vi "北控main.vi"() -> ()   [LabVIEW 2015]
uses:
  <vilib>/addons/database/Connection.llb/Conn ObjectReference.ctl
  <vilib>/addons/database/Auxilliary.llb/DB Tools Column Info.ctl
  <vilib>/addons/database/Auxilliary.llb/DB Tools DataTypes.ctl
  ModbusRTU/bin/Debug/Advantech.Adam.dll
  <vilib>/Instr/_visa.llb/VISA Flush IO Buffer Mask.ctl
  <vilib>/Utility/config.llb/Read Key (String).vi
  <vilib>/Utility/config.llb/Read Key (I32).vi
  <vilib>/Utility/config.llb/Read Key (Double).vi
  <vilib>/Instr/_visa.llb/VISA Configure Serial Port (Instr).vi
  <vilib>/Utility/config.llb/Write Key (String).vi
  <vilib>/Utility/config.llb/Write Key (I32).vi
  <vilib>/Utility/config.llb/Write Key (Double).vi
  <vilib>/regexp/Match Regular Expression.xnode
  <vilib>/addons/database/NI_Database_API.lvlib
  <vilib>/Utility/config.llb/NI_LVConfig.lvlib
panel:
  out "P1.0":dbl format="%#.3f"
  out "P2.0":dbl format="%#.3f"
  out "ISCOTCP":refnum<k5>
  in  "PressureCardID":i32=3
  out "adam串口正常":bool
  out "adamcom":refnum<k24>
  out "adammodbus":refnum<k24>
  out "TCPSuspend":bool
  in  "Adjust":dbl
  in  "WaterSeperation1.0":dbl
  in  "OilSeperation1.0":dbl
  out "OilValueCal":bool
  out "WaterValueCal":bool
  in  "PreOilValue":dbl
  in  "PreWaterValue":dbl
  out "ICControl":refnum<k7>
  out "YRDTCP":refnum<k5>
  out "Mettler VISA":refnum<visa-resource-name> caption="VISA资源名称输出"
  out "Mettler串口正常":bool
  in  "column information":T1=[{"column name"="RecordingTime", "data type"=enum."String", "size"=50, "allow null?"=TRUE}, {"column name"="CumulativeOilProduction", "data type"=enum."Double (DBL)", "size"=0, "allow null?"=TRUE}, {"column name"="CumulativeWaterProduction", "data type"=enum."Double (DBL)", "size"=0, "allow null?"=TRUE}, {"column name"="BalanceValue", "data type"=enum."Double (DBL)", "size"=0, "allow null?"=TRUE}, {"column name"="DifferencialPressure", "data type"=enum."Double (DBL)", "size"=0, "allow null?"=TRUE}, {"column name"="Pressure1", "data type"=enum."Double (DBL)", "size"=0, "allow null?"=TRUE}, {"column name"="Pressure2", "data type"=enum."Double (DBL)", "size"=0, "allow null?"=TRUE}, {"column name"="CPPOuterPre", "data type"=enum."Double (DBL)", "size"=0, "allow null?"=TRUE}, {"column name"="CPPTracePre", "data type"=enum."Double (DBL)", "size"=0, "allow null?"=TRUE}, {"column name"="CPPCurrentVol", "data type"=enum."Double (DBL)", "size"=0, "allow null?"=TRUE}, {"column name"="CPPInnerPre", "data type"=enum."Double (DBL)", "size"=0, "allow null?"=TRUE}, {"column name"="FlowSetpointA", "data type"=enum."Double (DBL)", "size"=0, "allow null?"=TRUE}, {"column name"="PressureSetpointA", "data type"=enum."Double (DBL)", "size"=0, "allow null?"=TRUE}, {"column name"="FlowRateA", "data type"=enum."Double (DBL)", "size"=0, "allow null?"=TRUE}, {"column name"="PressuerA", "data type"=enum."Double (DBL)", "size"=0, "allow null?"=TRUE}, {"column name"="FlowSetpointB", "data type"=enum."Double (DBL)", "size"=0, "allow null?"=TRUE}, {"column name"="PressureSetpointB", "data type"=enum."Double (DBL)", "size"=0, "allow null?"=TRUE}, {"column name"="FlowRateB", "data type"=enum."Double (DBL)", "size"=0, "allow null?"=TRUE}, {"column name"="PressuerB", "data type"=enum."Double (DBL)", "size"=0, "allow null?"=TRUE}, {"column name"="InspectionItem", "data type"=enum."String", "size"=0, "allow null?"=TRUE}, {"column name"="WellNumber", "data type"=enum."String", "size"=0, "allow null?"=TRUE}, {"column name"="DateofExperiment", "data type"=enum."String", "size"=0, "allow null?"=TRUE}, {"column name"="NumberofSample", "data type"=enum."String", "size"=0, "allow null?"=TRUE}, {"column name"="LithologicalCharacter ", "data type"=enum."String", "size"=0, "allow null?"=TRUE}, {"column name"="ExperimentalTemperature ", "data type"=enum."String", "size"=0, "allow null?"=TRUE}, {"column name"="SimulatedOilViscosity ", "data type"=enum."String", "size"=0, "allow null?"=TRUE}, {"column name"="InjectionWaterViscosity", "data type"=enum."String", "size"=0, "allow null?"=TRUE}, {"column name"="LengthofRockSample", "data type"=enum."String", "size"=0, "allow null?"=TRUE}, {"column name"="PoreVolume ", "data type"=enum."String", "size"=0, "allow null?"=TRUE}, {"column name"="CoreDepth ", "data type"=enum."String", "size"=0, "allow null?"=TRUE}, {"column name"="AirPermeability ", "data type"=enum."String", "size"=0, "allow null?"=TRUE}, {"column name"="SimulatedOilDensity", "data type"=enum."String", "size"=0, "allow null?"=TRUE}, {"column name"="InjectionWaterDensity", "data type"=enum."String", "size"=0, "allow null?"=TRUE}, {"column name"="RockSampleDiameter ", "data type"=enum."String", "size"=0, "allow null?"=TRUE}, {"column name"="Porosity", "data type"=enum."String", "size"=0, "allow null?"=TRUE}, {"column name"="InletPressure", "data type"=enum."String", "size"=0, "allow null?"=TRUE}, {"column name"="OutletPressure", "data type"=enum."String", "size"=0, "allow null?"=TRUE}, {"column name"="IrreducibleWaterSaturation", "data type"=enum."String", "size"=0, "allow null?"=TRUE}, {"column name"="SectionalArea", "data type"=enum."String", "size"=0, "allow null?"=TRUE}, {"column name"="VolumeOfRockSample", "data type"=enum."String", "size"=0, "allow null?"=TRUE}]
  out "Suspend":dbl
  out "Stop":dbl
  in  "选项卡控件":T4(tab)
  in  "压力校零":bool
  out "Pressure Setpoint B":dbl
  out "Flow Setpoint B":dbl
  out "Pressure Setpoint A":dbl
  out "Flow Setpoint A":dbl
  out "Pressure B":dbl
  out "Pressure A":dbl
  out "Flow Rate B":dbl
  out "Flow Rate A":dbl
  out "液罐 18":dbl(slide) scale=0.0..10.0
  out "液罐 26":dbl(slide) scale=0.0..10.0
  out "压差曲线":dbl(graph)
  out "压力曲线":cluster{"P1":dbl, "P2":dbl}(graph)
  out "布尔 157":bool
  in  "Mode Selection":u16(ring) items=["Oil-Water", "Oil-Gas"]
  out "液罐 9":dbl(slide) scale=0.0..10.0
  out "液罐 20":dbl(slide)=9.23076923076923 scale=0.0..10.0
  out "布尔 243":bool
  out "布尔 242":bool=TRUE
  in  "WaterValueCanlibration":bool
  out "WaterValue":dbl format="%#.3f"
  out "OilValue":dbl format="%#.3f"
  in  "OilValueCanlibration":bool
  out "DIF1":dbl format="%#.3g"
  out "P2(夹持器后端)":dbl format="%#.3f"
  out "液罐 17":dbl(slide) scale=0.0..10.0
  in  "DifPressure Canlibration":bool
  out "布尔 240":bool
  out "布尔 24":bool
  out "液罐 7":dbl(slide) scale=0.0..10.0
  out "布尔 6":bool
  out "液罐 6":dbl(slide) scale=0.0..10.0
  out "布尔 5":bool
  out "布尔 4":bool
  in  "btnExit":bool
  out "Weight":dbl format="%#.3f"
  out "布尔 8":bool
  out "布尔 25":bool
  out "液罐 10":dbl(slide) scale=0.0..10.0
  out "液罐 12":dbl(slide) scale=0.0..10.0
  out "液罐 13":dbl(slide) scale=0.0..10.0
  out "液罐 15":dbl(slide) scale=0.0..10.0
  out "液罐 16":dbl(slide) scale=0.0..10.0
  out "布尔 156":bool
  out "布尔 226":bool
  in  "灌泵":bool
  in  "打开跟踪泵":bool
  in  "SetDif(MPa)":dbl
  in  "SetPressure(MPa)":dbl
  in  "TraceMode":enum16{"TraceOuterPre", "TraceSetPre"}(ring)
  out "Suction":bool
  out "Drainage":bool
  in  "清泵":bool
  in  "关闭跟踪泵":bool
  out "CurrentVol(ml)":dbl format="%#.3g"
  out "InnerPre(MPa)":dbl format="%#.3g"
  out "TracePre(MPa)":dbl format="%#.3g"
  out "OuterPre(MPa)":dbl format="%#.3g"
  in  "SetVol(ml)":dbl
  in  "SafePre(MPa)":dbl
  out "P1(夹持器前端)":dbl format="%#.3f"
  in  "DocumentName":string
  in  "开始记录":bool
  in  "数值输入控件":dbl=2.0
  in  "文本下拉列表":u16(ring) items=["second", "minute"]
  out "Number":i32
  out "h":i64
  out "m":i32
  out "s":i32
  in  "停止记录":bool
  in  "暂停记录":bool
  in  "Change Document Name":bool
  in  "MettlerID":refnum<visa-resource-name>="COM11" caption="Mettler串口号"
  out "?":picture
  out "StartSaving":bool
  in  "ICImagingControl":refnum<k7>(container)
  out "数据库文件名":string
  out "DataBase":T5
  # "DataSaveConfiguration"
  # "DataSaveTimeInterval"
  # "psi"
  # "psi"
  # "psi"
  # "g"
  # "oil"
  # "oil"
  # "PMHP01"
  # "water"
  # "water"
  # "ml"
  # "Manual\n Pump"
  # "ml"
  # "BPV"
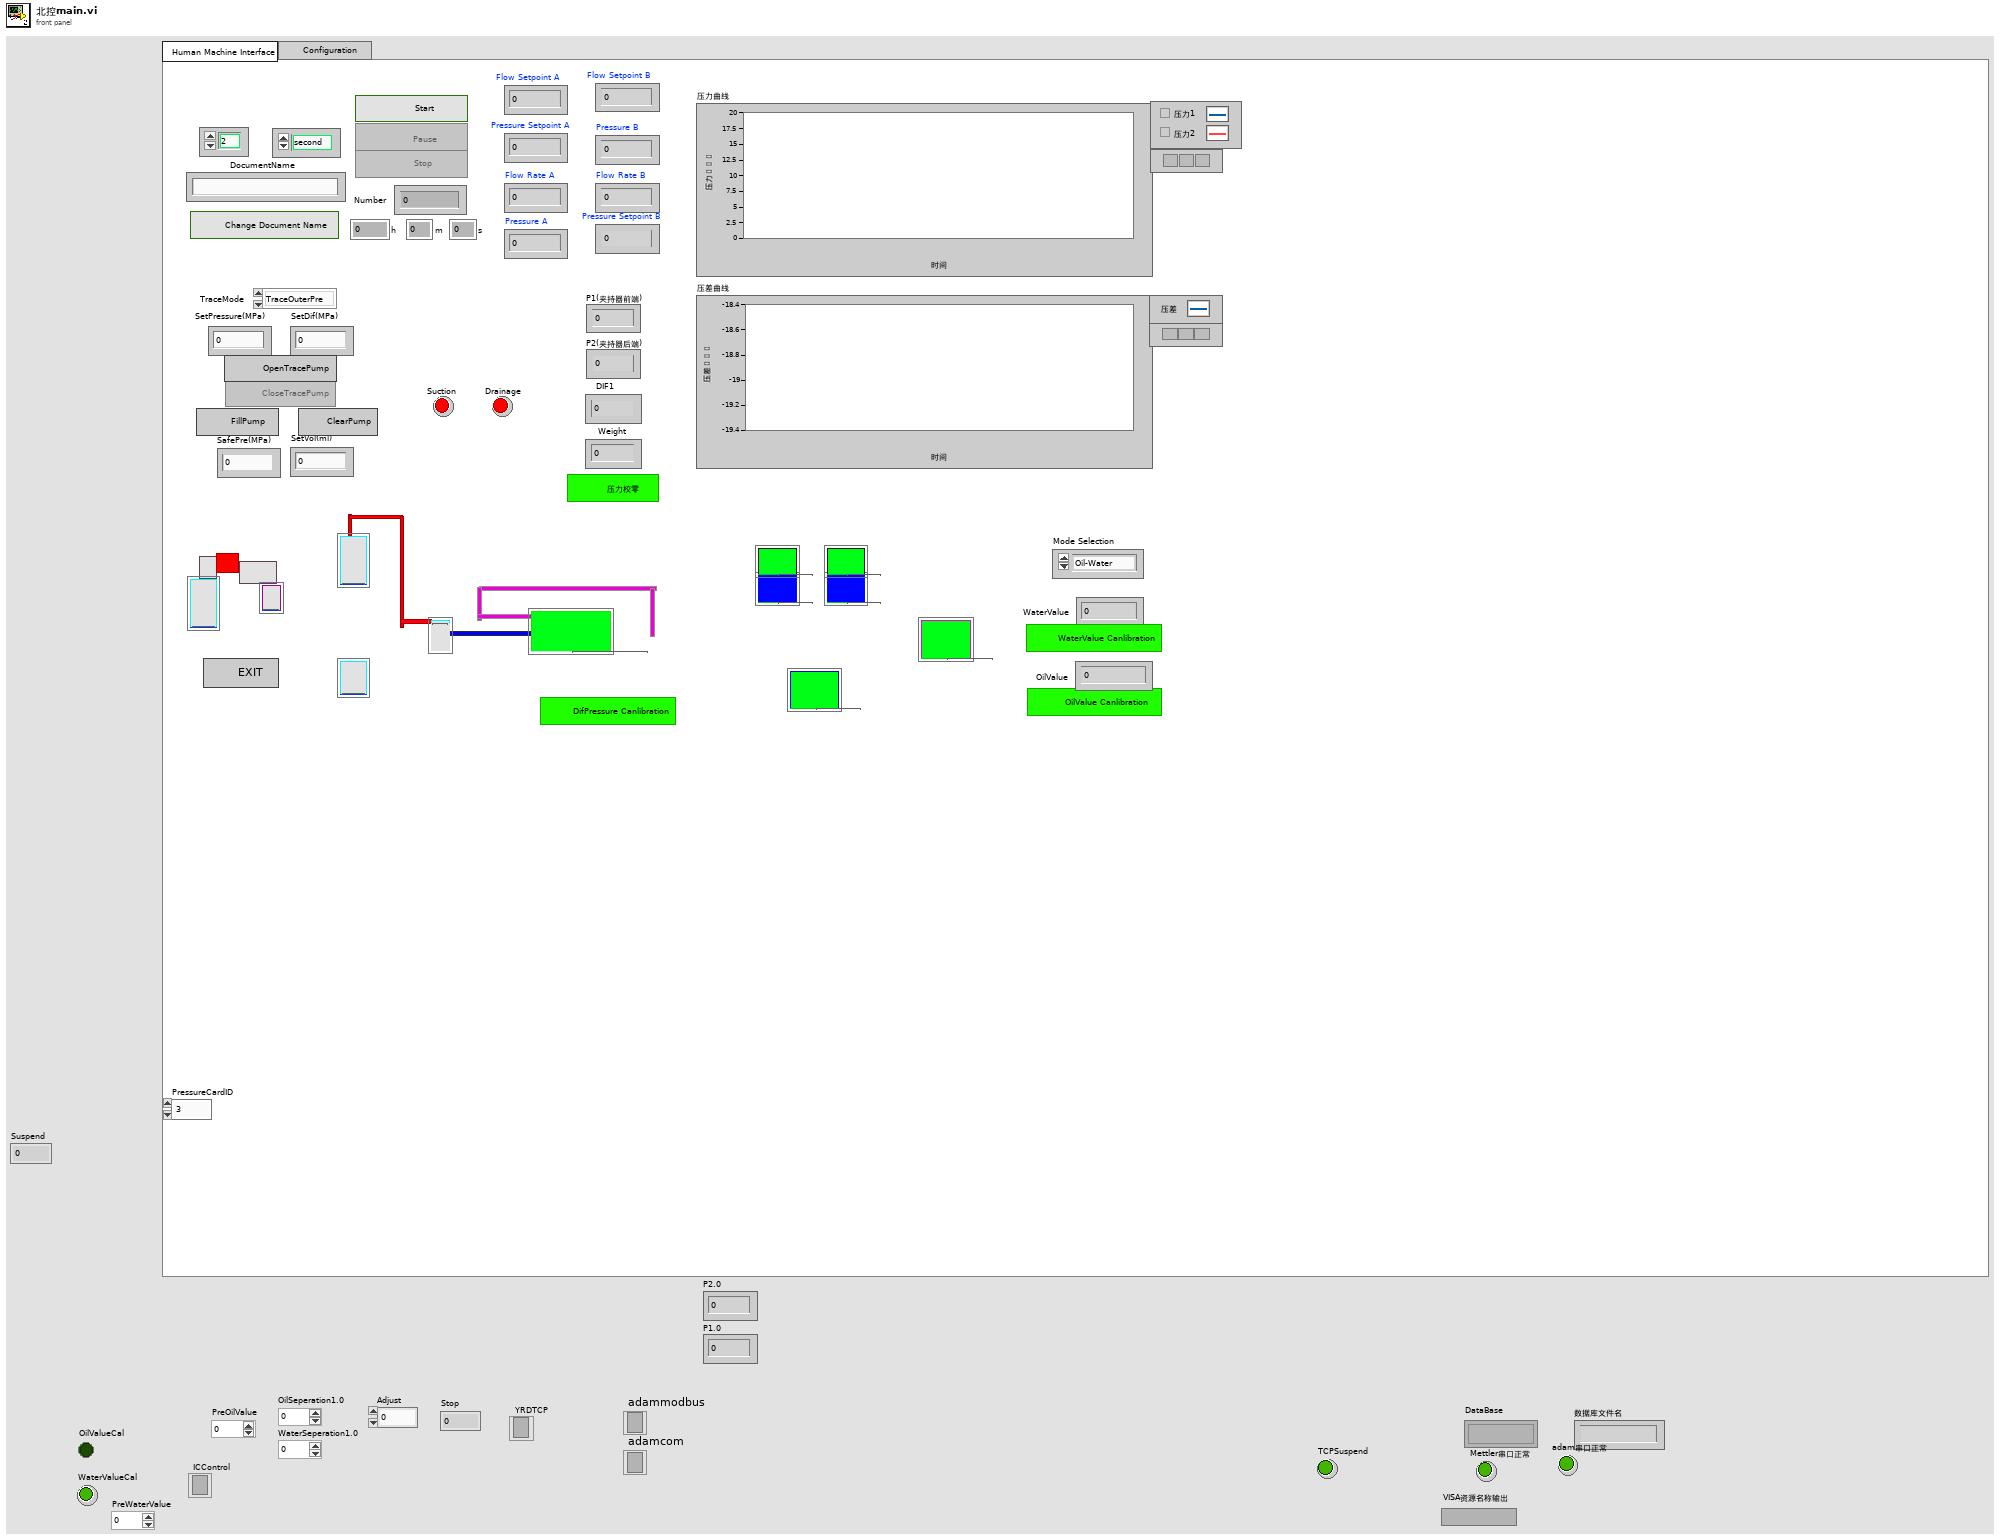
[diagram p1: front panel]
types:
  T1 = typedef "控件 1.ctl" = T2[]
  T2 = typedef "NI_Database_API.lvlib/DB Tools Column Info.ctl" = cluster{"column name":string, "data type":T3, "size":i32, "allow null?":bool}
  T3 = typedef "NI_Database_API.lvlib/DB Tools DataTypes.ctl" = enum16{"String", "Long (I32)", "Single (SGL)", "Double (DBL)", "Date/Time", "Binary"}
  T4 = enum32{" Human Machine Interface  ", "  Configuration            "}
  T5 = typedef "NI_Database_API.lvlib/Conn ObjectReference.ctl" = refnum<k1>
  T6 = enum8{"Enabled", "Disabled", "Disabled and Grayed Out"}
  T7 = typedef "NI_LVConfig.lvlib/Config Data RefNum.ctl" = refnum<k1>
  T8 = typedef "VISA Flush IO Buffer Mask.ctl" = u16
  T9 = cluster{string, "OilValue":dbl, "WaterValue":dbl, "Weight":dbl, "DIF1":dbl, "P1(夹持器前端)":dbl, "P2(夹持器后端)":dbl, "OuterPre(MPa)":dbl, "TracePre(MPa)":dbl, "CurrentVol(ml)":dbl, "InnerPre(MPa)":dbl, "Flow Setpoint A":dbl, "Pressure Setpoint A":dbl, "Flow Rate A":dbl, "Pressure A":dbl, "Flow Setpoint B":dbl, "Pressure Setpoint B":dbl, "Flow Rate B":dbl, "Pressure B":dbl}
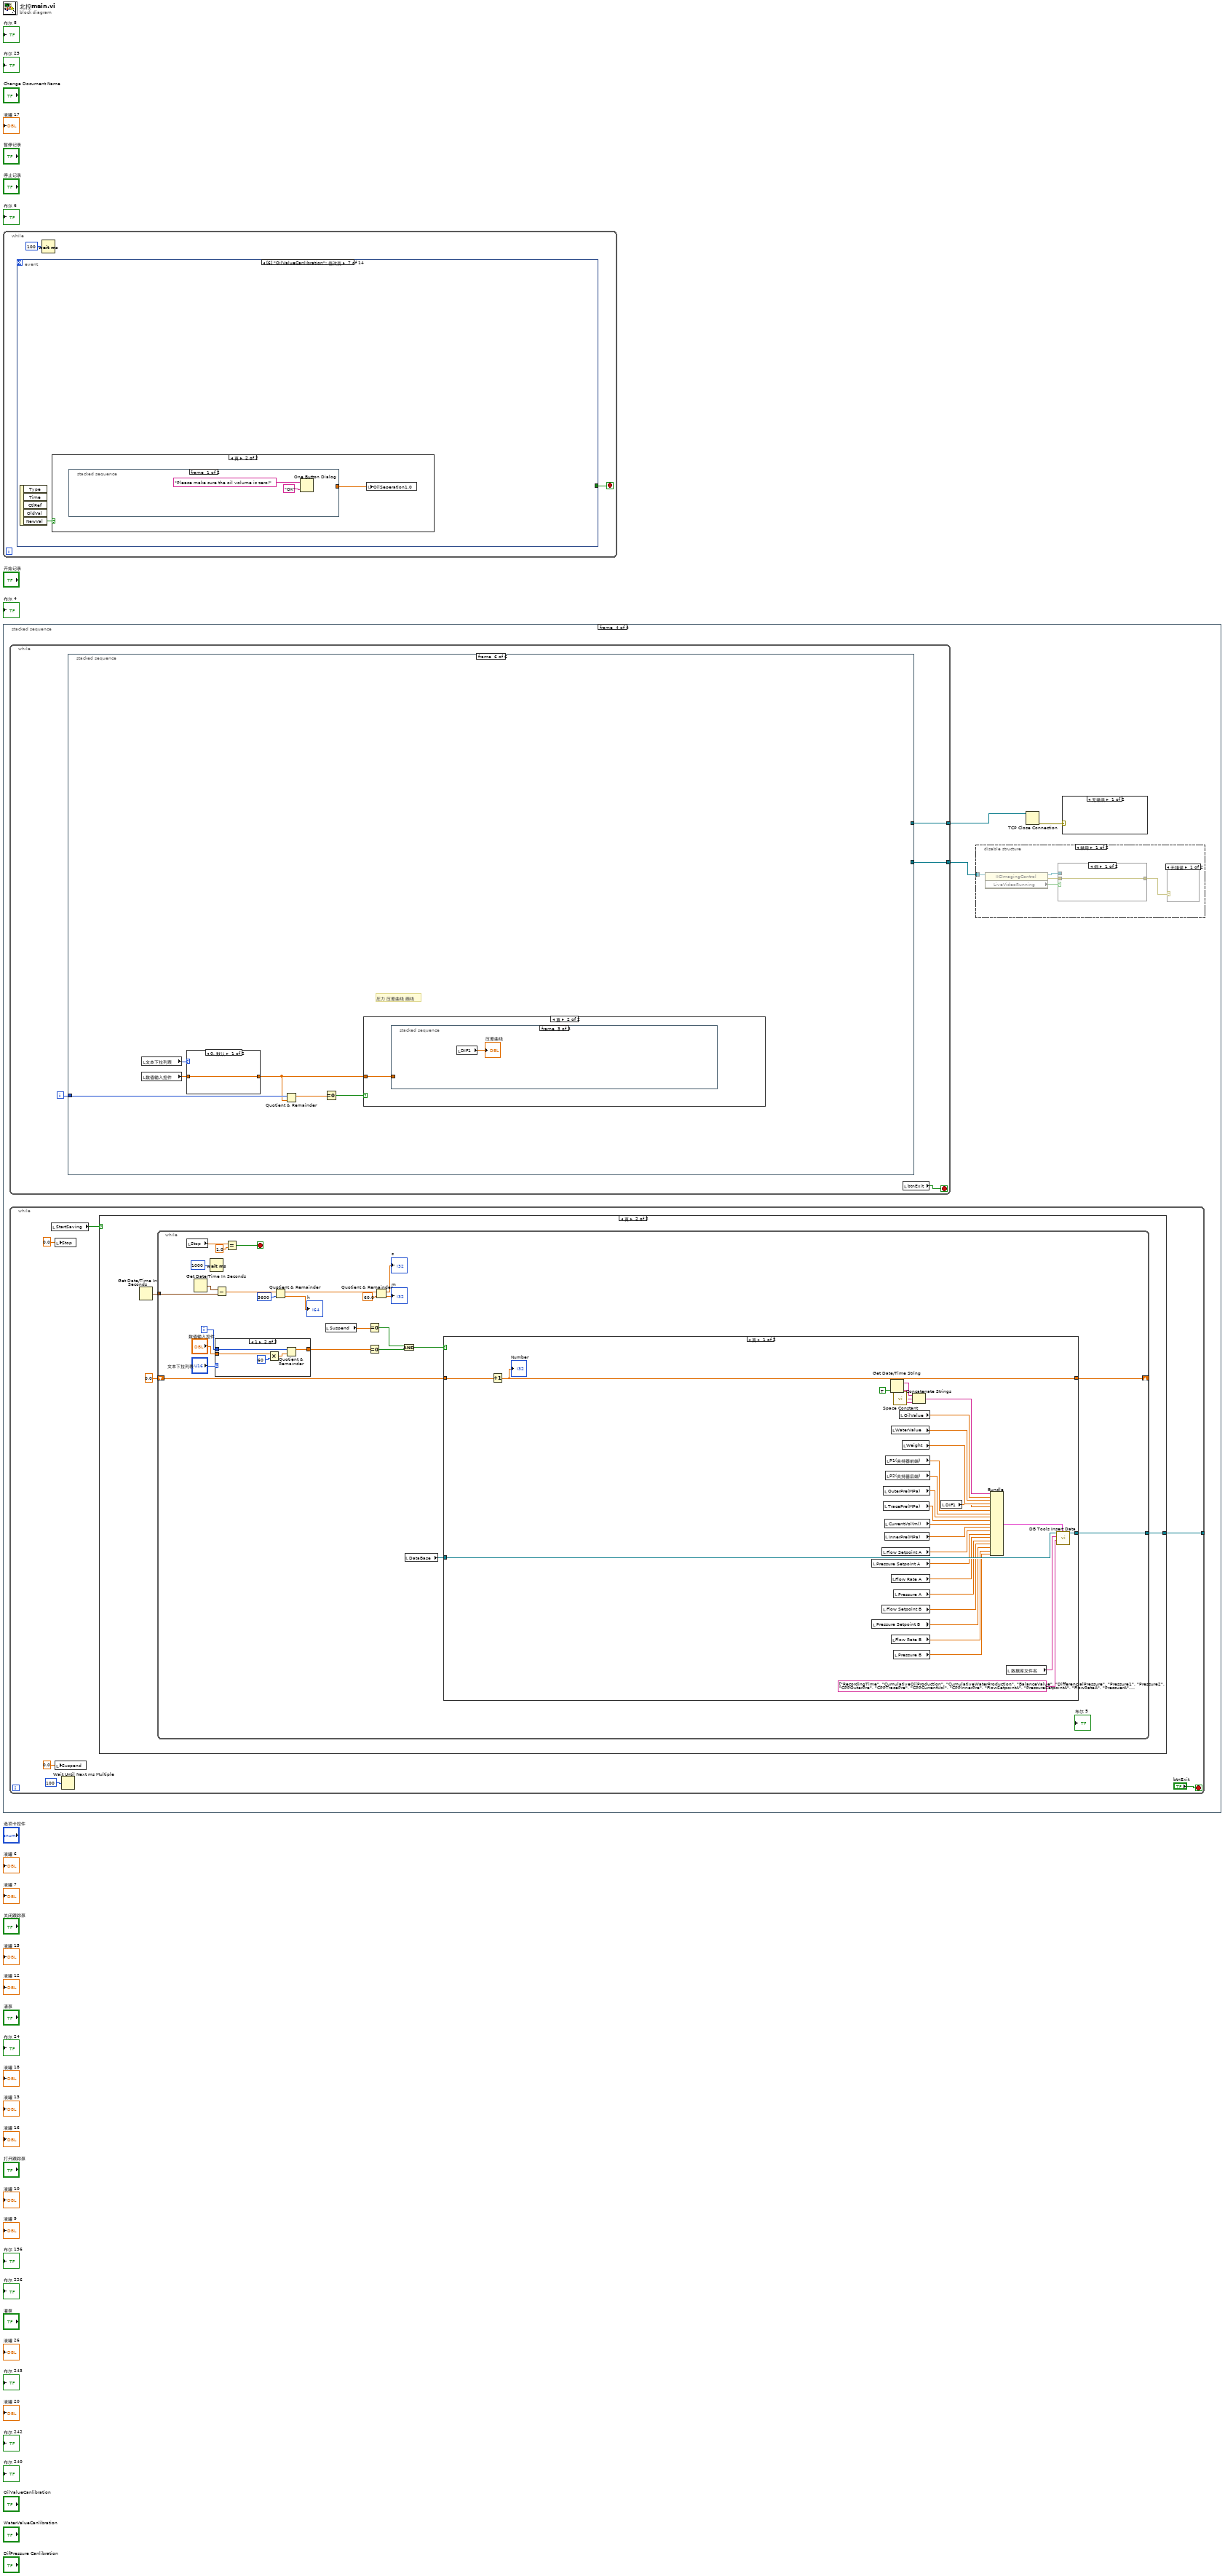
[diagram p0: block diagram]
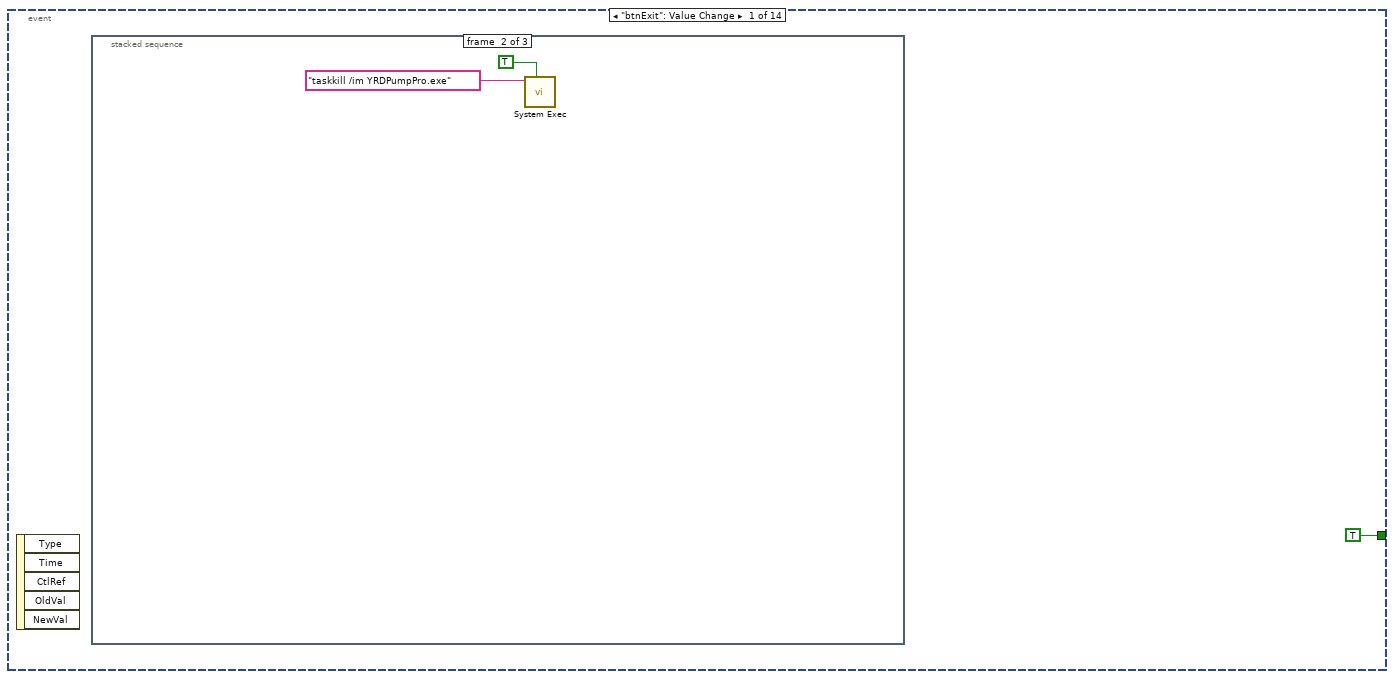
[diagram p2: hidden frame]
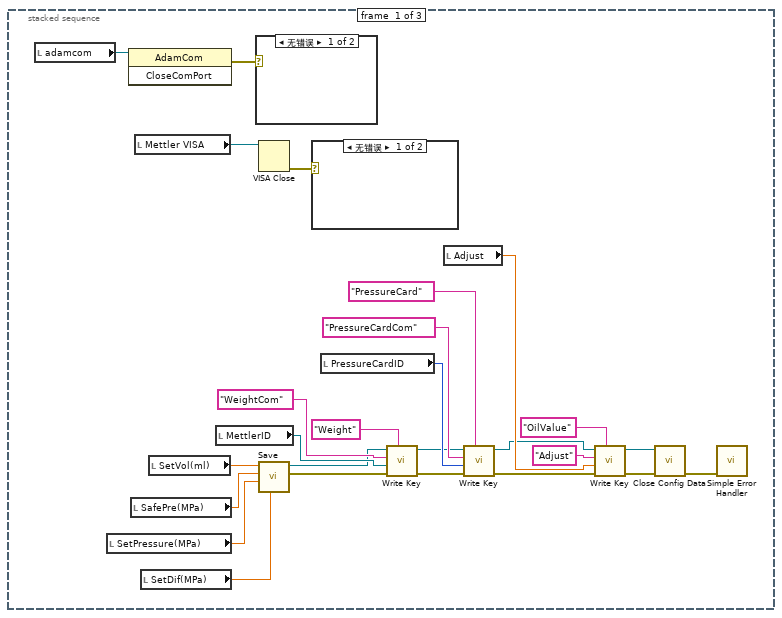
[diagram p3: hidden frame]
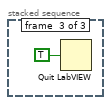
[diagram p6: hidden frame]
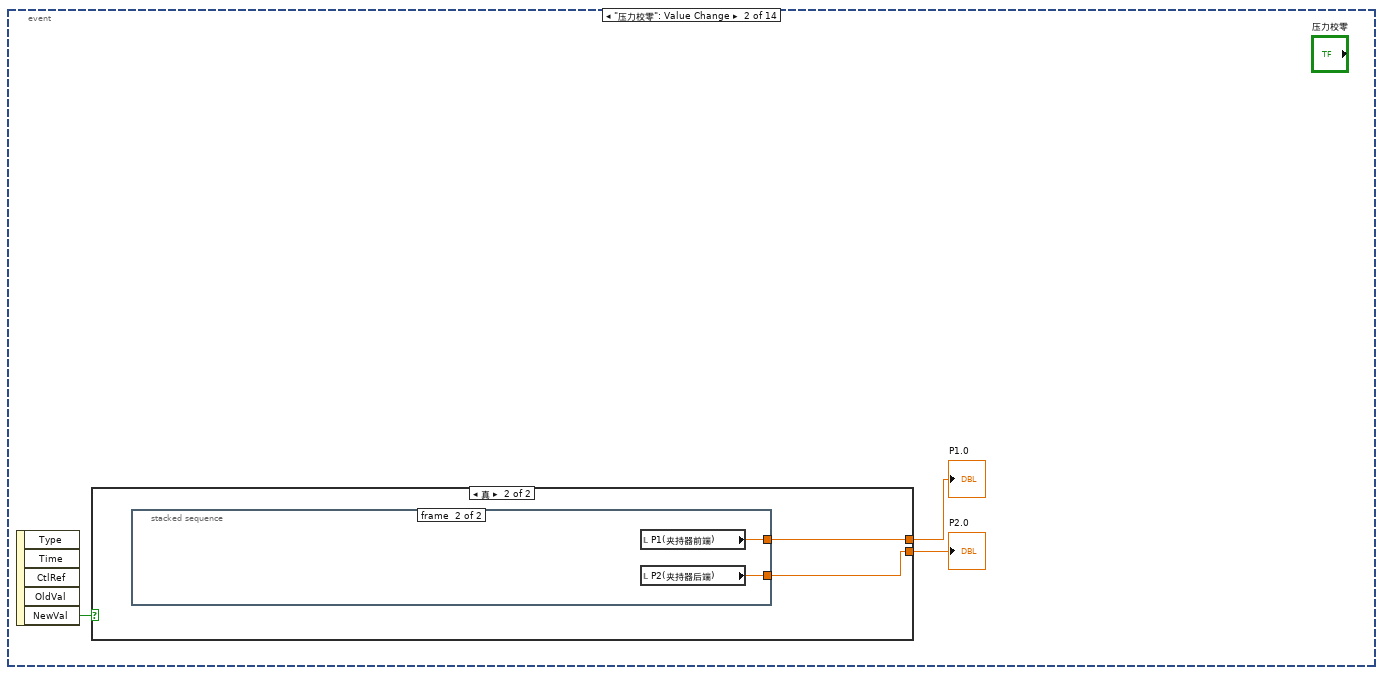
[diagram p7: hidden frame]
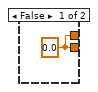
[diagram p8: hidden frame]
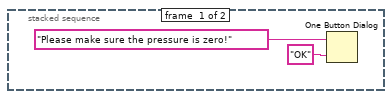
[diagram p9: hidden frame]
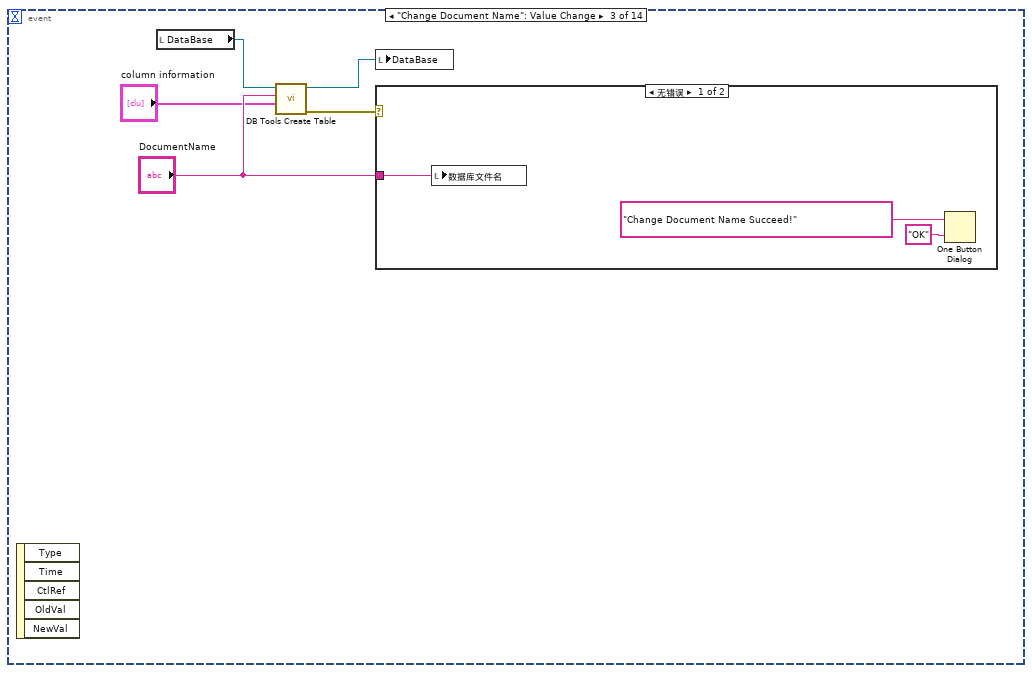
[diagram p10: hidden frame]
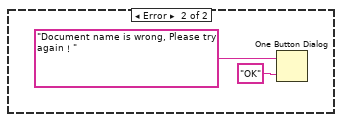
[diagram p11: hidden frame]
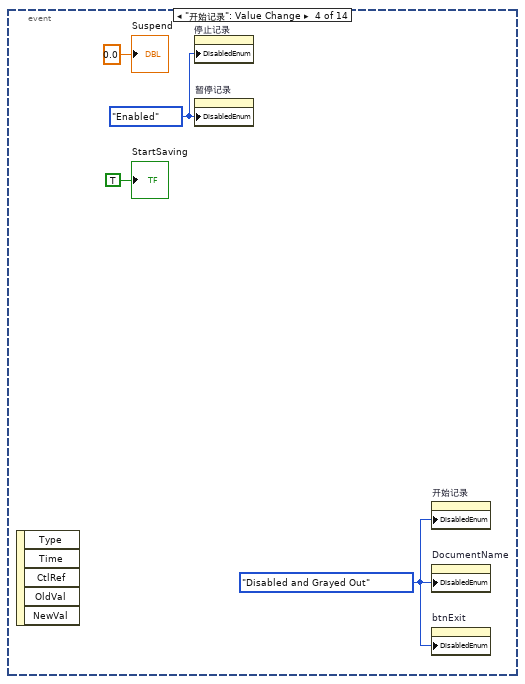
[diagram p12: hidden frame]
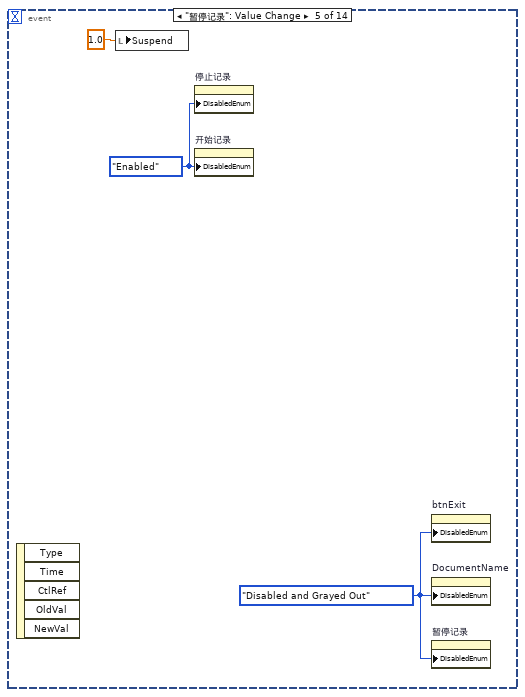
[diagram p13: hidden frame]
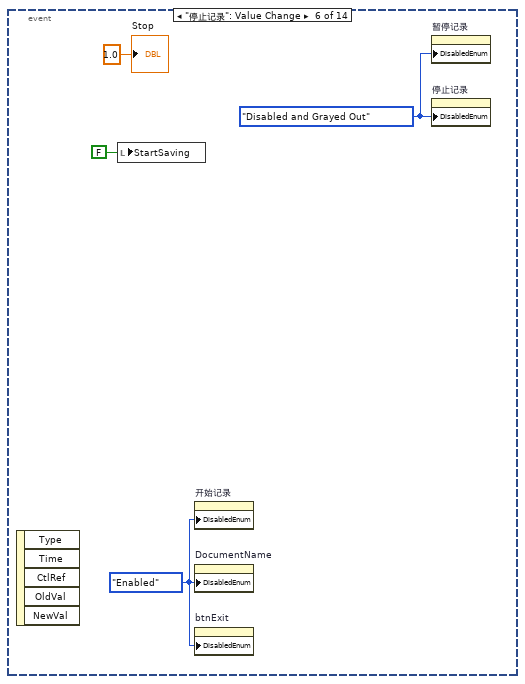
[diagram p14: hidden frame]
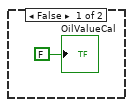
[diagram p15: hidden frame]
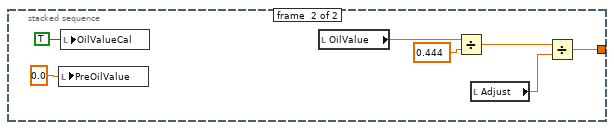
[diagram p16: hidden frame]
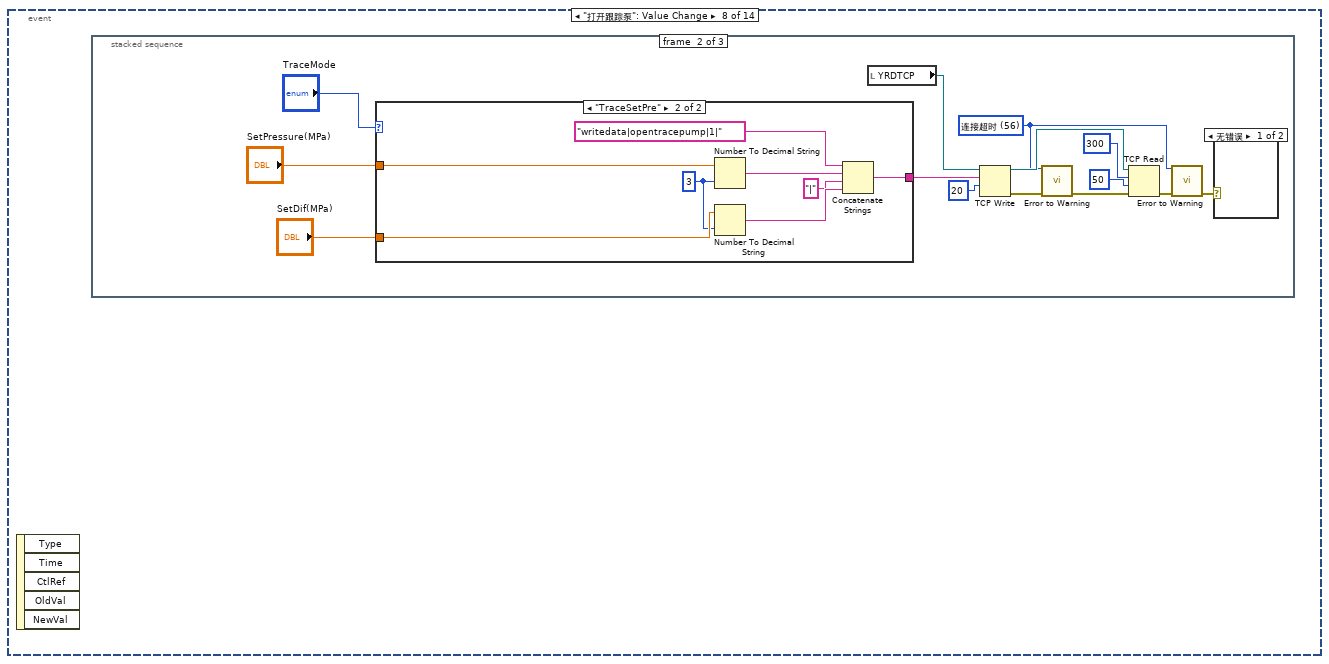
[diagram p17: hidden frame]
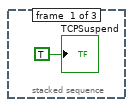
[diagram p18: hidden frame]
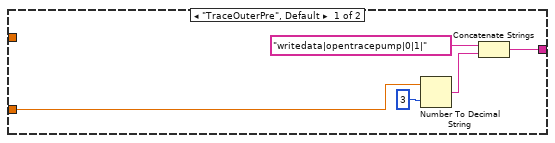
[diagram p20: hidden frame]
diagram:
  n1 = while {
    stop <- w1 stop-if-true
    n2 = event shown="[6] \"OilValueCanlibration\": 值改变" {
      selector: _ -> [_ _ _ _ _ _ _ _ _ _ _ _ _ _]
      dyn-events: _ -> [_ _ _ _ _ _ _ _ _ _ _ _ _ _]
      timeout: _ -> [_ _ _ _ _ _ _ _ _ _ _ _ _ _]
      tunnel: [TRUE _ _ _ _ _ _ _ _ _ _ _ _ _] -> w1
      event "btnExit": Value Change {
        n3 = event-data() -> ()  [unwired: 1 in, 5 out]
        n4 = stacked-sequence {
          frame #0 {
            n5 = local read "adamcom"() -> (w29:refnum<k24>)
            n6 = local read "SetPressure(MPa)"() -> (w26:dbl)
            n7 = invoke class="AdamCom" method="CloseComPort"(reference=w29) -> (error out=w4:errorcluster)  [unwired: 2 in, 2 out]
            n8 = local read "SafePre(MPa)"() -> (w28:dbl)
            n9 = local read "Mettler VISA"() -> (w6:refnum<visa-resource-name>)
            n10 = local read "SetDif(MPa)"() -> (w25:dbl)
            n11 = local read "SetVol(ml)"() -> (w27:dbl)
            n12 = local read "MettlerID"() -> (w11:refnum<visa-resource-name>)
            n13 = case shown="无错误" w4 {
              frame No Error {
              }
              frame Error {
              }
            }
            n14 = VISA Close(VISA resource name=w6) -> (error out=w5:errorcluster)  [unwired: 1 in]
            n15 = call "Save.vi"("SetDif(MPa)"=w25, "SetPressure(MPa)"=w26, "SafePre"=w28, "SetVol"=w27) -> ("error out"=w7:errorcluster, "refnum out"=w8:T7)  [unwired: 6 in]
            n16 = case shown="无错误" w5 {
              frame No Error {
              }
              frame Error {
              }
            }
            n17 = local read "PressureCardID"() -> (w15:i32)
            n18 = call-poly <vilib>:"Write Key.vi"("section"="Weight", "error in (no error)"=w7, "value"=w11, "key"="WeightCom", "refnum"=w8) -> ("error out"=w24:errorcluster, "refnum out"=w12:T7)  [unwired: 4 in, 1 out]
            n19 = local read "Adjust"() -> (w19:dbl)
            n20 = call-poly <vilib>:"Write Key.vi"("section"="PressureCard", "error in (no error)"=w24, "value"=w15, "key"="PressureCardCom", "refnum"=w12) -> ("error out"=w23:errorcluster, "refnum out"=w16:T7)  [unwired: 4 in, 1 out]
            n21 = call-poly <vilib>:"Write Key.vi"("section"="OilValue", "error in (no error)"=w23, "value"=w19, "key"="Adjust", "refnum"=w16) -> ("error out"=w22:errorcluster, "refnum out"=w21:T7)  [unwired: 4 in, 1 out]
            n22 = call <vilib>:"Close Config Data.vi"("error in (no error)"=w22, "refnum"=w21) -> ("error out"=w20:errorcluster)  [unwired: 1 in, 8 out]
            n23 = call <vilib>:"Simple Error Handler.vi"("error in (no error)"=w20) -> ()  [unwired: 1 in, 8 out]
          }
          frame #1 {
            n24 = call <vilib>:"System Exec.vi"("wait until completion? (T)"=TRUE, "command line"="taskkill /im YRDPumpPro.exe") -> ()  [unwired: 6 in, 4 out]
          }
          frame #2 {
            n25 = Quit LabVIEW(quit? (T)=TRUE ("退出？(T)")) -> ()
          }
        }
      }
      event "压力校零": Value Change {
        n26 = event-data() -> ("NewVal"=w35:bool)  [unwired: 1 in, 4 out]
        n27 = case shown="真" w35 {
          tunnel: [w36 w38] -> w34
          tunnel: [w36 w37] -> w33
          frame False {
            w36 = 0.0 ("P2(夹持器后端)")
          }
          frame True {
            n28 = stacked-sequence {
              tunnel: [_ w42] -> w38
              tunnel: [_ w41] -> w37
              frame #0 {
                n29 = One Button Dialog(message="Please make sure the pressure is zero!" ("消息"), button name ("OK")="OK" ("按钮名称（“确定”）")) -> ()  [unwired: 1 out]
              }
              frame #1 {
                n30 = local read "P1(夹持器前端)"() -> (w41:dbl)
                n31 = local read "P2(夹持器后端)"() -> (w42:dbl)
              }
            }
          }
        }
        "P2.0" <- w34
        "P1.0" <- w33
      }
      event "Change Document Name": Value Change {
        n32 = event-data() -> ()  [unwired: 1 in, 5 out]
        n33 = local read "DataBase"() -> (w47:T5)
        n34 = call <vilib>:"DB Tools Create Table.vi"("column information"="column information", "table"="DocumentName", "connection reference"=w47) -> ("error out"=w45:errorcluster, "connection reference out"=w46:T5)  [unwired: 5 in]
        n35 = local write "DataBase"(w46) -> ()
        n36 = case shown="无错误" w45 {
          tunnel: "DocumentName" -> [w50 _]
          frame No Error {
            n37 = local write "数据库文件名"(w50) -> ()
            n38 = One Button Dialog(message="Change Document Name Succeed!" ("消息"), button name ("OK")="OK" ("按钮名称（“确定”）")) -> ()  [unwired: 1 out]
          }
          frame Error {
            n39 = One Button Dialog(message="Document name is wrong, Please try again！" ("消息"), button name ("OK")="OK" ("按钮名称（“确定”）")) -> ()  [unwired: 1 out]
          }
        }
      }
      event "开始记录": Value Change {
        w53 = T6."Enabled" ("禁用")
        w54 = T6."Disabled and Grayed Out" ("禁用")
        n40 = event-data() -> ()  [unwired: 1 in, 5 out]
        n41 = property on="停止记录" class="Bool (严格)"("DisabledEnum"=w53) -> ()  [unwired: 2 in, 2 out]
        n42 = property on="暂停记录" class="Bool"("DisabledEnum"=w53) -> ()  [unwired: 2 in, 2 out]
        n43 = property on="开始记录" class="Bool (严格)"("DisabledEnum"=w54) -> ()  [unwired: 2 in, 2 out]
        n44 = property on="DocumentName" class="Str"("DisabledEnum"=w54) -> ()  [unwired: 2 in, 2 out]
        n45 = property on="btnExit" class="Bool (严格)"("DisabledEnum"=w54) -> ()  [unwired: 2 in, 2 out]
        "StartSaving" <- TRUE ("StartSaving")
        "Suspend" <- 0.0 ("Suspend")
      }
      event "暂停记录": Value Change {
        w57 = T6."Enabled" ("禁用")
        w58 = T6."Disabled and Grayed Out" ("禁用")
        n46 = event-data() -> ()  [unwired: 1 in, 5 out]
        n47 = local write "Suspend"(1.0 ("Suspend")) -> ()
        n48 = property on="停止记录" class="Bool (严格)"("DisabledEnum"=w57) -> ()  [unwired: 2 in, 2 out]
        n49 = property on="开始记录" class="Bool (严格)"("DisabledEnum"=w57) -> ()  [unwired: 2 in, 2 out]
        n50 = property on="btnExit" class="Bool (严格)"("DisabledEnum"=w58) -> ()  [unwired: 2 in, 2 out]
        n51 = property on="DocumentName" class="Str"("DisabledEnum"=w58) -> ()  [unwired: 2 in, 2 out]
        n52 = property on="暂停记录" class="Bool"("DisabledEnum"=w58) -> ()  [unwired: 2 in, 2 out]
      }
      event "停止记录": Value Change {
        w62 = T6."Enabled" ("禁用")
        w61 = T6."Disabled and Grayed Out" ("禁用")
        n53 = event-data() -> ()  [unwired: 1 in, 5 out]
        n54 = local write "StartSaving"(FALSE ("StartSaving")) -> ()
        n55 = property on="开始记录" class="Bool (严格)"("DisabledEnum"=w62) -> ()  [unwired: 2 in, 2 out]
        n56 = property on="DocumentName" class="Str"("DisabledEnum"=w62) -> ()  [unwired: 2 in, 2 out]
        n57 = property on="btnExit" class="Bool (严格)"("DisabledEnum"=w62) -> ()  [unwired: 2 in, 2 out]
        n58 = property on="暂停记录" class="Bool"("DisabledEnum"=w61) -> ()  [unwired: 2 in, 2 out]
        n59 = property on="停止记录" class="Bool (严格)"("DisabledEnum"=w61) -> ()  [unwired: 2 in, 2 out]
        "Stop" <- 1.0 ("Stop")
      }
      event "OilValueCanlibration": Value Change {
        n60 = event-data() -> ("NewVal"=w64:bool)  [unwired: 1 in, 4 out]
        n61 = case shown="真" w64 {
          frame False {
            "OilValueCal" <- FALSE ("OilValueCal")
          }
          frame True {
            n62 = stacked-sequence {
              tunnel: [_ w69] -> w66
              frame #0 {
                n63 = One Button Dialog(message="Please make sure the oil volume is zero!" ("消息"), button name ("OK")="OK" ("按钮名称（“确定”）")) -> ()  [unwired: 1 out]
              }
              frame #1 {
                n64 = local write "PreOilValue"(0.0 ("PreOilValue")) -> ()
                n65 = local write "OilValueCal"(TRUE ("OilValueCal")) -> ()
                n66 = local read "OilValue"() -> (w73:dbl)
                n67 = Divide(x=w73, y=0.444) -> (x/y=w71:dbl)
                n68 = local read "Adjust"() -> (w70:dbl)
                n69 = Divide(x=w71, y=w70) -> (x/y=w69:dbl)
              }
            }
            n70 = local write "OilSeperation1.0"(w66) -> ()
          }
        }
      }
      event "打开跟踪泵": Value Change {
        n71 = event-data() -> ()  [unwired: 1 in, 5 out]
        n72 = stacked-sequence {
          frame #0 {
            "TCPSuspend" <- TRUE ("TCPSuspend")
          }
          frame #1 {
            w81 = 56 items=["无错误", "参数错误", "内存已满", "超出区域", "文件结束", "文件已打开", "一般文件IO错误", "未找到文件", "文件权限错误", "磁盘已满", "路径副本", "打开过多文件", "未启用", "未找到资源文件", "无法添加资源", "未找到资源", "未找到图像", "图像内存错误", "画笔不存在", "配置错误类型", "配置未找到解析段", "配置解析错误", "配置内存错误", "错误外部代码格式", "错误外部代码偏移量", "外部代码不存在", "空窗口", "销毁窗口错误", "空菜单", "打印已中止", "错误打印记录", "打印驱动程序错误", "打印时窗口错误", "打印时内存错误", "打印对话框错误", "一般打印错误", "无效设备引用句柄", "设备未找到", "设备参数错误", "设备单位错误", "无法打开设备", "设备调用已中止", "一般错误", "用户已取消", "对象ID过低", "对象ID过高", "对象不在堆中", "未知的堆", "错误DefProc ID", "DefProc不在表格中", "范围外信息", "空方法", "未知信息", "不支持管理器调用", "错误地址", "连接过程中", "连接超时", "连接过程中", "不支持网络属性", "网络错误", "正在使用的地址", "系统缺少内存", "连接已中止", "连接已拒绝", "连接未建立", "连接已建立", "连接已关闭", "初始化错误（交互应用程序管理器）", "错误事件发生", "等待无约束事件发生处理程序", "事件发生队列溢出", "错误路径", "未发出信号量", "未识别类型（交互应用程序管理器）"] ("1st Error to Convert")
            n73 = case shown="\"TraceSetPre\"" "TraceMode" {
              tunnel: "SetPressure(MPa)" -> [_ w101]
              tunnel: [w93 w102] -> w90
              tunnel: "SetDif(MPa)" -> [w92 w99]
              frame "TraceOuterPre", Default {
                n74 = Number To Decimal String(number=w92, width (-)=i16 3 ("宽度(-)")) -> (decimal integer string=w95:string)
                n75 = Concatenate Strings("writedata|opentracepump|0|1|" ("字符串"), w95) -> (w93:string)
              }
              frame "TraceSetPre" {
                w96 = i16 3 ("宽度(-)")
                n76 = Number To Decimal String(number=w101, width (-)=w96) -> (decimal integer string=w100:string)
                n77 = Number To Decimal String(number=w99, width (-)=w96) -> (decimal integer string=w98:string)
                n78 = Concatenate Strings("writedata|opentracepump|1|" ("字符串"), w100, "|" ("字符串"), w98) -> (w102:string)
              }
            }
            n79 = local read "YRDTCP"() -> (w77:refnum<k5>)
            n80 = TCP Write(connection ID=w77, data in=w90, 9:20 ("超时毫秒(25000)")) -> (connection ID out=w89:refnum<k5>, error out=w86:errorcluster)  [unwired: 1 in, 1 out]
            n81 = call <vilib>:"Error to Warning.vi"("1st Error to Convert"=w81, "error in"=w86) -> ("warning out"=w84:errorcluster)  [unwired: 13 in]
            n82 = TCP Read(connection ID=w89, bytes to read=300 ("读取的字节"), error in (no error)=w84, 9:50 ("超时毫秒(25000)")) -> (error out=w83:errorcluster)  [unwired: 1 in, 2 out]
            n83 = call <vilib>:"Error to Warning.vi"("1st Error to Convert"=w81, "error in"=w83) -> ("warning out"=w82:errorcluster)  [unwired: 13 in]
            n84 = case shown="无错误" w82 {
              frame No Error {
              }
              frame Error {
              }
            }
          }
          frame #2 {
            w104 = T6."Disabled and Grayed Out" ("禁用")
            n85 = local write "TCPSuspend"(FALSE ("TCPSuspend")) -> ()
            n86 = property on="关闭跟踪泵" class="Bool"("DisabledEnum"=T6."Enabled" ("禁用")) -> ()  [unwired: 2 in, 2 out]
            n87 = property on="清泵" class="Bool"("DisabledEnum"=w104) -> ()  [unwired: 2 in, 2 out]
            n88 = property on="打开跟踪泵" class="Bool"("DisabledEnum"=w104) -> ()  [unwired: 2 in, 2 out]
            n89 = property on="灌泵" class="Bool"("DisabledEnum"=w104) -> ()  [unwired: 2 in, 2 out]
          }
        }
      }
      event "关闭跟踪泵": Value Change {
        n90 = event-data() -> ()  [unwired: 1 in, 5 out]
        n91 = stacked-sequence {
          frame #0 {
            n92 = local write "TCPSuspend"(TRUE ("TCPSuspend")) -> ()
          }
          frame #1 {
            w109 = 56 items=["无错误", "参数错误", "内存已满", "超出区域", "文件结束", "文件已打开", "一般文件IO错误", "未找到文件", "文件权限错误", "磁盘已满", "路径副本", "打开过多文件", "未启用", "未找到资源文件", "无法添加资源", "未找到资源", "未找到图像", "图像内存错误", "画笔不存在", "配置错误类型", "配置未找到解析段", "配置解析错误", "配置内存错误", "错误外部代码格式", "错误外部代码偏移量", "外部代码不存在", "空窗口", "销毁窗口错误", "空菜单", "打印已中止", "错误打印记录", "打印驱动程序错误", "打印时窗口错误", "打印时内存错误", "打印对话框错误", "一般打印错误", "无效设备引用句柄", "设备未找到", "设备参数错误", "设备单位错误", "无法打开设备", "设备调用已中止", "一般错误", "用户已取消", "对象ID过低", "对象ID过高", "对象不在堆中", "未知的堆", "错误DefProc ID", "DefProc不在表格中", "范围外信息", "空方法", "未知信息", "不支持管理器调用", "错误地址", "连接过程中", "连接超时", "连接过程中", "不支持网络属性", "网络错误", "正在使用的地址", "系统缺少内存", "连接已中止", "连接已拒绝", "连接未建立", "连接已建立", "连接已关闭", "初始化错误（交互应用程序管理器）", "错误事件发生", "等待无约束事件发生处理程序", "事件发生队列溢出", "错误路径", "未发出信号量", "未识别类型（交互应用程序管理器）"] ("1st Error to Convert")
            n93 = local read "YRDTCP"() -> (w108:refnum<k5>)
            n94 = TCP Write(connection ID=w108, data in="writedata|stoptracepump" ("数据输入"), 9:20 ("超时毫秒(25000)")) -> (connection ID out=w117:refnum<k5>, error out=w113:errorcluster)  [unwired: 1 in, 1 out]
            n95 = call <vilib>:"Error to Warning.vi"("1st Error to Convert"=w109, "error in"=w113) -> ("warning out"=w112:errorcluster)  [unwired: 13 in]
            n96 = TCP Read(connection ID=w117, bytes to read=300 ("读取的字节"), error in (no error)=w112, 9:50 ("超时毫秒(25000)")) -> (error out=w111:errorcluster)  [unwired: 1 in, 2 out]
            n97 = call <vilib>:"Error to Warning.vi"("1st Error to Convert"=w109, "error in"=w111) -> ("warning out"=w110:errorcluster)  [unwired: 13 in]
            n98 = case shown="无错误" w110 {
              frame No Error {
              }
              frame Error {
              }
            }
          }
          frame #2 {
            w119 = T6."Enabled" ("禁用")
            n99 = local write "TCPSuspend"(FALSE ("TCPSuspend")) -> ()
            n100 = property on="清泵" class="Bool"("DisabledEnum"=w119) -> ()  [unwired: 2 in, 2 out]
            n101 = property on="打开跟踪泵" class="Bool"("DisabledEnum"=w119) -> ()  [unwired: 2 in, 2 out]
            n102 = property on="灌泵" class="Bool"("DisabledEnum"=w119) -> ()  [unwired: 2 in, 2 out]
            n103 = property on="关闭跟踪泵" class="Bool"("DisabledEnum"=T6."Disabled and Grayed Out" ("禁用")) -> ()  [unwired: 2 in, 2 out]
          }
        }
      }
      event "清泵": Value Change {
        n104 = event-data() -> ()  [unwired: 1 in, 5 out]
        n105 = stacked-sequence {
          frame #0 {
            n106 = local write "TCPSuspend"(TRUE ("TCPSuspend")) -> ()
          }
          frame #1 {
            w124 = 56 items=["无错误", "参数错误", "内存已满", "超出区域", "文件结束", "文件已打开", "一般文件IO错误", "未找到文件", "文件权限错误", "磁盘已满", "路径副本", "打开过多文件", "未启用", "未找到资源文件", "无法添加资源", "未找到资源", "未找到图像", "图像内存错误", "画笔不存在", "配置错误类型", "配置未找到解析段", "配置解析错误", "配置内存错误", "错误外部代码格式", "错误外部代码偏移量", "外部代码不存在", "空窗口", "销毁窗口错误", "空菜单", "打印已中止", "错误打印记录", "打印驱动程序错误", "打印时窗口错误", "打印时内存错误", "打印对话框错误", "一般打印错误", "无效设备引用句柄", "设备未找到", "设备参数错误", "设备单位错误", "无法打开设备", "设备调用已中止", "一般错误", "用户已取消", "对象ID过低", "对象ID过高", "对象不在堆中", "未知的堆", "错误DefProc ID", "DefProc不在表格中", "范围外信息", "空方法", "未知信息", "不支持管理器调用", "错误地址", "连接过程中", "连接超时", "连接过程中", "不支持网络属性", "网络错误", "正在使用的地址", "系统缺少内存", "连接已中止", "连接已拒绝", "连接未建立", "连接已建立", "连接已关闭", "初始化错误（交互应用程序管理器）", "错误事件发生", "等待无约束事件发生处理程序", "事件发生队列溢出", "错误路径", "未发出信号量", "未识别类型（交互应用程序管理器）"] ("1st Error to Convert")
            n107 = local read "YRDTCP"() -> (w123:refnum<k5>)
            n108 = TCP Write(connection ID=w123, data in="writedata|clearpump" ("数据输入"), 9:20 ("超时毫秒(25000)")) -> (connection ID out=w132:refnum<k5>, error out=w128:errorcluster)  [unwired: 1 in, 1 out]
            n109 = call <vilib>:"Error to Warning.vi"("1st Error to Convert"=w124, "error in"=w128) -> ("warning out"=w127:errorcluster)  [unwired: 13 in]
            n110 = TCP Read(connection ID=w132, bytes to read=300 ("读取的字节"), error in (no error)=w127, 9:50 ("超时毫秒(25000)")) -> (error out=w126:errorcluster)  [unwired: 1 in, 2 out]
            n111 = call <vilib>:"Error to Warning.vi"("1st Error to Convert"=w124, "error in"=w126) -> ("warning out"=w125:errorcluster)  [unwired: 13 in]
            n112 = case shown="无错误" w125 {
              frame No Error {
              }
              frame Error {
              }
            }
          }
          frame #2 {
            w134 = T6."Disabled and Grayed Out" ("禁用")
            n113 = local write "TCPSuspend"(FALSE ("TCPSuspend")) -> ()
            n114 = property on="关闭跟踪泵" class="Bool"("DisabledEnum"=T6."Enabled" ("禁用")) -> ()  [unwired: 2 in, 2 out]
            n115 = property on="清泵" class="Bool"("DisabledEnum"=w134) -> ()  [unwired: 2 in, 2 out]
            n116 = property on="打开跟踪泵" class="Bool"("DisabledEnum"=w134) -> ()  [unwired: 2 in, 2 out]
            n117 = property on="灌泵" class="Bool"("DisabledEnum"=w134) -> ()  [unwired: 2 in, 2 out]
          }
        }
      }
      event "灌泵": Value Change {
        n118 = event-data() -> ()  [unwired: 1 in, 5 out]
        n119 = stacked-sequence {
          frame #0 {
            n120 = local write "TCPSuspend"(TRUE ("TCPSuspend")) -> ()
          }
          frame #1 {
            w139 = 56 items=["无错误", "参数错误", "内存已满", "超出区域", "文件结束", "文件已打开", "一般文件IO错误", "未找到文件", "文件权限错误", "磁盘已满", "路径副本", "打开过多文件", "未启用", "未找到资源文件", "无法添加资源", "未找到资源", "未找到图像", "图像内存错误", "画笔不存在", "配置错误类型", "配置未找到解析段", "配置解析错误", "配置内存错误", "错误外部代码格式", "错误外部代码偏移量", "外部代码不存在", "空窗口", "销毁窗口错误", "空菜单", "打印已中止", "错误打印记录", "打印驱动程序错误", "打印时窗口错误", "打印时内存错误", "打印对话框错误", "一般打印错误", "无效设备引用句柄", "设备未找到", "设备参数错误", "设备单位错误", "无法打开设备", "设备调用已中止", "一般错误", "用户已取消", "对象ID过低", "对象ID过高", "对象不在堆中", "未知的堆", "错误DefProc ID", "DefProc不在表格中", "范围外信息", "空方法", "未知信息", "不支持管理器调用", "错误地址", "连接过程中", "连接超时", "连接过程中", "不支持网络属性", "网络错误", "正在使用的地址", "系统缺少内存", "连接已中止", "连接已拒绝", "连接未建立", "连接已建立", "连接已关闭", "初始化错误（交互应用程序管理器）", "错误事件发生", "等待无约束事件发生处理程序", "事件发生队列溢出", "错误路径", "未发出信号量", "未识别类型（交互应用程序管理器）"] ("1st Error to Convert")
            n121 = local read "YRDTCP"() -> (w138:refnum<k5>)
            n122 = TCP Write(connection ID=w138, data in="writedata|fullpump" ("数据输入"), 9:20 ("超时毫秒(25000)")) -> (connection ID out=w147:refnum<k5>, error out=w144:errorcluster)  [unwired: 1 in, 1 out]
            n123 = call <vilib>:"Error to Warning.vi"("1st Error to Convert"=w139, "error in"=w144) -> ("warning out"=w142:errorcluster)  [unwired: 13 in]
            n124 = TCP Read(connection ID=w147, bytes to read=300 ("读取的字节"), error in (no error)=w142, 9:50 ("超时毫秒(25000)")) -> (error out=w141:errorcluster)  [unwired: 1 in, 2 out]
            n125 = call <vilib>:"Error to Warning.vi"("1st Error to Convert"=w139, "error in"=w141) -> ("warning out"=w140:errorcluster)  [unwired: 13 in]
            n126 = case shown="无错误" w140 {
              frame No Error {
              }
              frame Error {
              }
            }
          }
          frame #2 {
            w149 = T6."Disabled and Grayed Out" ("禁用")
            n127 = local write "TCPSuspend"(FALSE ("TCPSuspend")) -> ()
            n128 = property on="关闭跟踪泵" class="Bool"("DisabledEnum"=T6."Enabled" ("禁用")) -> ()  [unwired: 2 in, 2 out]
            n129 = property on="清泵" class="Bool"("DisabledEnum"=w149) -> ()  [unwired: 2 in, 2 out]
            n130 = property on="灌泵" class="Bool"("DisabledEnum"=w149) -> ()  [unwired: 2 in, 2 out]
            n131 = property on="打开跟踪泵" class="Bool"("DisabledEnum"=w149) -> ()  [unwired: 2 in, 2 out]
          }
        }
      }
      event "SafePre(MPa)": Value Change {
        n132 = event-data() -> ()  [unwired: 1 in, 5 out]
        n133 = stacked-sequence {
          frame #0 {
            n134 = local write "TCPSuspend"(TRUE ("TCPSuspend")) -> ()
          }
          frame #1 {
            w155 = 56 items=["无错误", "参数错误", "内存已满", "超出区域", "文件结束", "文件已打开", "一般文件IO错误", "未找到文件", "文件权限错误", "磁盘已满", "路径副本", "打开过多文件", "未启用", "未找到资源文件", "无法添加资源", "未找到资源", "未找到图像", "图像内存错误", "画笔不存在", "配置错误类型", "配置未找到解析段", "配置解析错误", "配置内存错误", "错误外部代码格式", "错误外部代码偏移量", "外部代码不存在", "空窗口", "销毁窗口错误", "空菜单", "打印已中止", "错误打印记录", "打印驱动程序错误", "打印时窗口错误", "打印时内存错误", "打印对话框错误", "一般打印错误", "无效设备引用句柄", "设备未找到", "设备参数错误", "设备单位错误", "无法打开设备", "设备调用已中止", "一般错误", "用户已取消", "对象ID过低", "对象ID过高", "对象不在堆中", "未知的堆", "错误DefProc ID", "DefProc不在表格中", "范围外信息", "空方法", "未知信息", "不支持管理器调用", "错误地址", "连接过程中", "连接超时", "连接过程中", "不支持网络属性", "网络错误", "正在使用的地址", "系统缺少内存", "连接已中止", "连接已拒绝", "连接未建立", "连接已建立", "连接已关闭", "初始化错误（交互应用程序管理器）", "错误事件发生", "等待无约束事件发生处理程序", "事件发生队列溢出", "错误路径", "未发出信号量", "未识别类型（交互应用程序管理器）"] ("1st Error to Convert")
            n135 = Number To Decimal String(number="SafePre(MPa)") -> (decimal integer string=w163:string)  [unwired: 1 in]
            n136 = local read "YRDTCP"() -> (w154:refnum<k5>)
            n137 = Concatenate Strings("writedata|setsafepress|" ("数据输入"), w163) -> (w161:string)
            n138 = TCP Write(connection ID=w154, data in=w161, 9:20 ("超时毫秒(25000)")) -> (connection ID out=w166:refnum<k5>, error out=w160:errorcluster)  [unwired: 1 in, 1 out]
            n139 = call <vilib>:"Error to Warning.vi"("1st Error to Convert"=w155, "error in"=w160) -> ("warning out"=w158:errorcluster)  [unwired: 13 in]
            n140 = TCP Read(connection ID=w166, bytes to read=300 ("读取的字节"), error in (no error)=w158, 9:50 ("超时毫秒(25000)")) -> (error out=w157:errorcluster)  [unwired: 1 in, 2 out]
            n141 = call <vilib>:"Error to Warning.vi"("1st Error to Convert"=w155, "error in"=w157) -> ("warning out"=w156:errorcluster)  [unwired: 13 in]
            n142 = case shown="无错误" w156 {
              frame No Error {
              }
              frame Error {
              }
            }
          }
          frame #2 {
            n143 = local write "TCPSuspend"(FALSE ("TCPSuspend")) -> ()
          }
        }
      }
      event "SetVol(ml)": Value Change {
        n144 = event-data() -> ()  [unwired: 1 in, 5 out]
        n145 = stacked-sequence {
          frame #0 {
            n146 = local write "TCPSuspend"(TRUE ("TCPSuspend")) -> ()
          }
          frame #1 {
            w171 = 56 items=["无错误", "参数错误", "内存已满", "超出区域", "文件结束", "文件已打开", "一般文件IO错误", "未找到文件", "文件权限错误", "磁盘已满", "路径副本", "打开过多文件", "未启用", "未找到资源文件", "无法添加资源", "未找到资源", "未找到图像", "图像内存错误", "画笔不存在", "配置错误类型", "配置未找到解析段", "配置解析错误", "配置内存错误", "错误外部代码格式", "错误外部代码偏移量", "外部代码不存在", "空窗口", "销毁窗口错误", "空菜单", "打印已中止", "错误打印记录", "打印驱动程序错误", "打印时窗口错误", "打印时内存错误", "打印对话框错误", "一般打印错误", "无效设备引用句柄", "设备未找到", "设备参数错误", "设备单位错误", "无法打开设备", "设备调用已中止", "一般错误", "用户已取消", "对象ID过低", "对象ID过高", "对象不在堆中", "未知的堆", "错误DefProc ID", "DefProc不在表格中", "范围外信息", "空方法", "未知信息", "不支持管理器调用", "错误地址", "连接过程中", "连接超时", "连接过程中", "不支持网络属性", "网络错误", "正在使用的地址", "系统缺少内存", "连接已中止", "连接已拒绝", "连接未建立", "连接已建立", "连接已关闭", "初始化错误（交互应用程序管理器）", "错误事件发生", "等待无约束事件发生处理程序", "事件发生队列溢出", "错误路径", "未发出信号量", "未识别类型（交互应用程序管理器）"] ("1st Error to Convert")
            n147 = Number To Fractional String(number="SetVol(ml)") -> (F-format string=w179:string)  [unwired: 3 in]
            n148 = local read "YRDTCP"() -> (w170:refnum<k5>)
            n149 = Concatenate Strings("writedata|setabsorborrelfluw|" ("数据输入"), w179) -> (w177:string)
            n150 = TCP Write(connection ID=w170, data in=w177, 9:20 ("超时毫秒(25000)")) -> (connection ID out=w182:refnum<k5>, error out=w176:errorcluster)  [unwired: 1 in, 1 out]
            n151 = call <vilib>:"Error to Warning.vi"("1st Error to Convert"=w171, "error in"=w176) -> ("warning out"=w174:errorcluster)  [unwired: 13 in]
            n152 = TCP Read(connection ID=w182, bytes to read=300 ("读取的字节"), error in (no error)=w174, 9:50 ("超时毫秒(25000)")) -> (error out=w173:errorcluster)  [unwired: 1 in, 2 out]
            n153 = call <vilib>:"Error to Warning.vi"("1st Error to Convert"=w171, "error in"=w173) -> ("warning out"=w172:errorcluster)  [unwired: 13 in]
            n154 = case shown="无错误" w172 {
              frame No Error {
              }
              frame Error {
              }
            }
          }
          frame #2 {
            n155 = local write "TCPSuspend"(FALSE ("TCPSuspend")) -> ()
          }
        }
      }
      event "WaterValueCanlibration": Value Change {
        n156 = event-data() -> ("NewVal"=w184:bool)  [unwired: 1 in, 4 out]
        n157 = case shown="真" w184 {
          frame False {
            "WaterValueCal" <- FALSE ("WaterValueCal")
          }
          frame True {
            n158 = stacked-sequence {
              tunnel: [_ w192] -> w186
              frame #0 {
                n159 = One Button Dialog(message="Please make sure the oil volume is zero!" ("消息"), button name ("OK")="OK" ("按钮名称（“确定”）")) -> ()  [unwired: 1 out]
              }
              frame #1 {
                n160 = local write "PreWaterValue"(0.0 ("PreOilValue")) -> ()
                n161 = local write "WaterValueCal"(TRUE ("OilValueCal")) -> ()
                n162 = local read "WaterValue"() -> (w189:dbl)
                n163 = Divide(x=w189, y=0.444) -> (x/y=w194:dbl)
                n164 = local read "Adjust"() -> (w193:dbl)
                n165 = Divide(x=w194, y=w193) -> (x/y=w192:dbl)
              }
            }
            n166 = local write "WaterSeperation1.0"(w186) -> ()
          }
        }
      }
    }
    n167 = Wait (ms)(milliseconds to wait=u32 100 ("等待时间（毫秒）")) -> ()  [unwired: 1 out]
  }
  n168 = stacked-sequence {
    frame #0 {
      n169 = call "登录对话框.vi"() -> ("显示文件名"=w198:string, "access out"=→"DataBase":T5)  [unwired: 1 in]
      "数据库文件名" <- w198
      n170 = local write "DocumentName"(w198) -> ()
      n171 = String To Path(string="C:\\Program Files\\SmartAutoBeiKong") -> (path=w196:path)
      n172 = call <vilib>:"Check if File or Folder Exists.vi"("path"=w196) -> ("file or folder exists?"=w197:bool)  [unwired: 8 in, 2 out]
      n173 = case shown="真" w197 {
        tunnel: w196 -> [w201 _]
        frame False {
          n174 = Create Folder(path (use dialog)=w201) -> ()  [unwired: 2 in, 3 out]
        }
        frame True {
          n175 = call "YRDParaRead.vi"("字符串"="C:\\Program Files\\SmartAutoBeiKong\\config.ini") -> ("错误输出"=w213:errorcluster, "SetPressure"=w206:dbl, "SetDif"=w207:dbl, "引用句柄输出"=w211:T7, "SetVol"=w205:dbl, "SafePre"=w208:dbl)  [unwired: 5 in]
          n176 = local write "SetPressure(MPa)"(w206) -> ()
          n177 = local write "SafePre(MPa)"(w208) -> ()
          n178 = local write "SetDif(MPa)"(w207) -> ()
          n179 = local write "SetVol(ml)"(w205) -> ()
          n180 = call-poly <vilib>:"Read Key.vi"("section"="Weight", "error in (no error)"=w213, "key"="WeightCom", "refnum"=w211) -> ("error out"=w216:errorcluster, "value"=w204:string, "refnum out"=w215:T7)  [unwired: 4 in, 1 out]
          n181 = local write "MettlerID"(w204) -> ()
          n182 = call-poly <vilib>:"Read Key.vi"("section"="PressureCard", "error in (no error)"=w216, "key"="PressureCardCom", "refnum"=w215) -> ("error out"=w223:errorcluster, "value"=w203:i32, "refnum out"=w219:T7)  [unwired: 4 in, 1 out]
          n183 = local write "PressureCardID"(w203) -> ()
          n184 = call-poly <vilib>:"Read Key.vi"("section"="OilValue", "error in (no error)"=w223, "key"="Adjust", "refnum"=w219) -> ("error out"=w224:errorcluster, "value"=w202:dbl, "refnum out"=w222:T7)  [unwired: 4 in, 1 out]
          n185 = local write "Adjust"(w202) -> ()
          n186 = call <vilib>:"Close Config Data.vi"("error in (no error)"=w224, "refnum"=w222) -> ("error out"=w214:errorcluster)  [unwired: 1 in, 8 out]
          n187 = call <vilib>:"Simple Error Handler.vi"("error in (no error)"=w214) -> ()  [unwired: 1 in, 8 out]
        }
      }
    }
    frame #1 {
      n188 = Wait (ms)(milliseconds to wait=u32 5000 ("等待时间（毫秒）")) -> ()  [unwired: 1 out]
      n189 = call <vilib>:"Application Directory.vi"() -> ("Application Directory"=w229:path)
      n190 = Path To String(path=w229) -> (string=w232:string)
      n191 = Concatenate Strings(w232, "\\Debug\\YRDPumpPro.exe" ("字符串")) -> (w230:string)
      n192 = call <vilib>:"System Exec.vi"("wait until completion? (T)"=FALSE, "command line"="C:\\Program Files\\注入泵\\注入泵.exe") -> ()  [unwired: 6 in, 4 out]
      n193 = call <vilib>:"System Exec.vi"("wait until completion? (T)"=FALSE, "command line"=w230) -> ()  [unwired: 6 in, 4 out]
    }
    frame #2 {
      w251 = FALSE ("WaterValueCal")
      w261 = T8 16 items=["清空接收缓冲区"=16, "向设备写入传输缓冲区"=32, "清空接收缓冲区（无I/O）"=64, "清空传输缓冲区"=128] ("Mask")
      w264 = T6."Enabled" ("禁用")
      w263 = T6."Disabled and Grayed Out" ("禁用")
      # "Mettler天平  串口打开"
      # "YRD泵  TCP端口打开"
      # "ISCO泵 TCP端口 打开"
      # "视频采集开始"
      # "adam压力采集（2路） 串口打开"
      n194 = local write "WaterValueCal"(w251) -> ()
      n195 = local write "OilValueCal"(w251) -> ()
      n196 = property on="停止记录" class="Bool (严格)"("DisabledEnum"=w263) -> ()  [unwired: 2 in, 2 out]
      n197 = property on="暂停记录" class="Bool"("DisabledEnum"=w263) -> ()  [unwired: 2 in, 2 out]
      n198 = TCP Open Connection(address="127.0.0.1" ("地址"), remote port or service name=u16 8000 ("Port")) -> (connection ID=→"YRDTCP":refnum<k5>, error out=w252:errorcluster)  [unwired: 3 in]
      n199 = TCP Open Connection(address="127.0.0.1" ("地址"), remote port or service name=u16 19000 ("Port")) -> (connection ID=→"ISCOTCP":refnum<k5>, error out=w240:errorcluster)  [unwired: 3 in]
      n200 = call "adam_init.vi"("Address"=1, "COM Port"="PressureCardID") -> ("错误输出"=w247:errorcluster, "com"=→"adamcom":refnum<k24>, "modbus"=→"adammodbus":refnum<k24>)  [unwired: 7 in]
      n201 = call-poly "VISA Configure Serial Port"("VISA resource name"="MettlerID", "baud rate (9600)"=u32 9600, "data bits (8)"=u16 8) -> ("VISA resource name out"=w259:refnum<visa-resource-name>, "error out"=w262:errorcluster)  [unwired: 11 in]
      n202 = case shown="错误" w247 {
        tunnel: [TRUE ("adam串口正常") FALSE ("adam串口正常")] -> w246
        frame No Error {
        }
        frame Error {
          n203 = One Button Dialog(message="Open Pressure Card Failed!" ("消息"), button name ("OK")="OK" ("按钮名称（“确定”）")) -> ()  [unwired: 1 out]
        }
      }
      "adam串口正常" <- w246
      n204 = call <vilib>:"Application Directory.vi"() -> ("Application Directory"=w236:path)
      n205 = Path To String(path=w236) -> (string=w237:string)
      n206 = case shown="错误" w262 {
        tunnel: [TRUE ("串口错误") FALSE ("串口错误")] -> w245
        frame No Error {
        }
        frame Error {
          n207 = One Button Dialog(message="Open Mettler Failed!" ("消息"), button name ("OK")="OK" ("按钮名称（“确定”）")) -> ()  [unwired: 1 out]
        }
      }
      "Mettler串口正常" <- w245
      n208 = case shown="错误" w240 {
        frame No Error {
        }
        frame Error {
          n209 = One Button Dialog(message="创建侦听失败，请检查isco泵" ("消息"), button name ("OK")="OK" ("按钮名称（“确定”）")) -> ()  [unwired: 1 out]
        }
      }
      n210 = VISA Flush I/O Buffer(VISA resource name=w259, mask (16)=w261, error in (no error)=w262) -> (VISA resource name out=→"Mettler VISA":refnum<visa-resource-name>)  [unwired: 1 out]
      n211 = case shown="错误" w252 {
        frame No Error {
        }
        frame Error {
          n212 = One Button Dialog(message="Open YRD Failed!" ("消息"), button name ("OK")="OK" ("按钮名称（“确定”）")) -> ()  [unwired: 1 out]
        }
      }
      n213 = Concatenate Strings(w237, "\\data\\image device.dat" ("字符串")) -> (w239:string)
      n214 = String To Path(string=w239) -> (path=w234:path)
      n215 = call "ic初始化.vi"("路径"=w234, "自动化引用句柄输入"="ICImagingControl") -> ("自动化引用句柄输入 2"=→"ICControl":refnum<k7>)  [unwired: 9 in]
      n216 = property on="btnExit" class="Bool (严格)"("DisabledEnum"=w264) -> ()  [unwired: 2 in, 2 out]
      n217 = property on="DocumentName" class="Str"("DisabledEnum"=w264) -> ()  [unwired: 2 in, 2 out]
      n218 = property on="开始记录" class="Bool (严格)"("DisabledEnum"=w264) -> ()  [unwired: 2 in, 2 out]
    }
    frame #3 {
      n219 = while {
        tunnel: [w291] -> w279
        tunnel: [w289] -> w278
        i -> [w290]
        stop <- w292 stop-if-true
        n220 = stacked-sequence {
          tunnel: [_ _ w455 _ _ _] -> w291
          tunnel: w290 -> [_ _ _ w503 _ w529]
          tunnel: [_ _ _ w502 _ _] -> w289
          frame #0 {
            # "天平串口  读重量"
            n221 = local read "Mettler串口正常"() -> (w293:bool)
            n222 = case shown="真" w293 {
              frame False {
              }
              frame True {
                n223 = local read "Mettler VISA"() -> (w303:refnum<visa-resource-name>)
                n224 = Concatenate Strings("SI" ("写入缓冲区"), "\r", "\n") -> (w307:string)
                n225 = VISA Write(VISA resource name=w303, write buffer=w307) -> (VISA resource name out=w310:refnum<visa-resource-name>, error out=w308:errorcluster)  [unwired: 1 in, 1 out]
                n226 = disable-structure shown="启用" {
                  disable-tunnel: [w316 _] -> w309
                  disable-tunnel: w308 -> [w314 _]
                  frame Disabled {
                    n227 = call <userlib>:"Wait (ms)__ogtk.vi"("error in (no error)"=w314, "milliseconds to wait"=u32 100) -> ("error out"=w316:errorcluster)  [unwired: 8 in, 1 out]
                  }
                  frame Enabled {
                  }
                }
                n228 = property class="Instr"(reference=w310, error in=w309) -> (reference out=w312:refnum<visa-resource-name>, error out=w311:errorcluster, "Serial Settings:Number of Bytes at Serial Port"=w313:u32)
                n229 = VISA Read(VISA resource name=w312, byte count=w313, error in (no error)=w311) -> (read buffer=w296:string)  [unwired: 3 out]
                n230 = xnode "匹配正则表达式"("输入字符串"=w296, "正则表达式"="\\d+\\.\\d+") -> ("匹配之前"=w302:string, "所有匹配"=w297:string)  [unwired: 4 in, 3 out]
                n231 = String Length(string=w302) -> (length=w298:i32)
                n232 = Fract/Exp String To Number(string=w297) -> (number=w301:dbl)  [unwired: 3 in, 1 out]
                n233 = Decrement(x=w298) -> (x-1=w299:i32)
                n234 = String Subset(string=w302, offset (0)=w299) -> (substring=w300:string)  [unwired: 1 in]
                n235 = case shown="\"-\"" w300 {
                  tunnel: w301 -> [w317 w319]
                  tunnel: [w317 w320] -> w294
                  frame "+", Default {
                  }
                  frame "-" {
                    n236 = Subtract(x=0.0, y=w319) -> (x-y=w320:dbl)
                  }
                }
                "Weight" <- w294
              }
            }
          }
          frame #1 {
            # "压力串口  读两个压力值"
            n237 = local read "adam串口正常"() -> (w432:bool)
            n238 = case shown="真" w432 {
              frame False {
              }
              frame True {
                n239 = local read "adammodbus"() -> (w453:refnum<k24>)
                n240 = invoke class="Modbus" method="ReadHoldingRegs"(reference=w453, "i_iStartIndex"=2, "i_iTotalPoint"=2) -> ("o_iData"=w450:i32[])  [unwired: 3 in, 5 out]
                n241 = Index Array(array=w450, index #1=0 ("索引"), index #2=1 ("索引")) -> (element #1=w446:i32, element #2=w439:i32)
                n242 = Multiply(x=70.0, y=145.0) -> (x*y=w440:dbl)
                n243 = Multiply(x=70.0, y=145.0) -> (x*y=w445:dbl)
                n244 = call "压力量程转换为工程量.vi"("量程"=w440, "数值输入"=w439) -> ("数值输出"=w435:dbl)  [unwired: 1 in]
                n245 = call "压力量程转换为工程量.vi"("量程"=w445, "数值输入"=w446) -> ("数值输出"=w438:dbl)  [unwired: 1 in]
                n246 = local read "P1.0"() -> (w434:dbl)
                n247 = local read "P2.0"() -> (w437:dbl)
                n248 = Subtract(x=w435, y=w434) -> (x-y=w433:dbl)
                "P1(夹持器前端)" <- w433
                n249 = Subtract(x=w438, y=w437) -> (x-y=w436:dbl)
                "P2(夹持器后端)" <- w436
                n250 = Subtract(x=w433, y=w436) -> (x-y=→"DIF1":dbl)
              }
            }
          }
          frame #2 {
            # "YRD 泵相关值读取"
            n251 = local read "TCPSuspend"() -> (w456:bool)
            n252 = local read "YRDTCP"() -> (w454:refnum<k5>)
            n253 = case shown="假" w456 {
              tunnel: [w459 w470] -> w455
              tunnel: w454 -> [w458 w470]
              frame False {
                n254 = call "TCPR.vi"("connection ID"=w458) -> ("吸液阀状态"=w469:i32, "内部压力"=→"InnerPre(MPa)":dbl, "外部压力"=→"OuterPre(MPa)":dbl, "连接ID输出"=w459:refnum<k5>, "跟踪压力"=→"TracePre(MPa)":dbl, "错误输出"=w457:errorcluster, "当前泵容量"=→"CurrentVol(ml)":dbl, "排液阀状态"=w464:i32)  [unwired: 1 in]
                n255 = Equal To 0?(x=w469) -> (x = 0?=w468:bool)
                n256 = case shown="无错误" w457 {
                  frame No Error {
                  }
                  frame Error {
                  }
                }
                n257 = Equal To 0?(x=w464) -> (x = 0?=w465:bool)
                n258 = Not(x=w468) -> (.not. x?=→"Suction":bool)
                n259 = Not(x=w465) -> (.not. x?=→"Drainage":bool)
              }
              frame True {
              }
            }
          }
          frame #3 {
            # "图像处理 读取有水值比例"
            n260 = call <vilib>:"Application Directory.vi"() -> ("Application Directory"=w486:path)
            n261 = Path To String(path=w486) -> (string=w485:string)
            n262 = local read "ICControl"() -> (w482:refnum<k7>)
            n263 = Concatenate Strings(w485, "\\data\\Tem.bmp" ("字符串")) -> (w483:string)
            n264 = String To Path(string=w483) -> (path=w497:path)
            n265 = call "IC_Grab_Picture.vi"("ICImagingControl In"=w482) -> ("ICImagingControl Out"=w502:refnum<k7>, "Picture Out"=→"?":picture, "Error Out"=w495:errorcluster)  [unwired: 1 in, 1 out]
            n266 = invoke class="Pict" method="Export Image"(error in=w495, "File Type"=enum32{"BMP", "EPS", "EMF", "PICT"}."BMP" ("文件类型"), "Target"=enum32{"File", "Clipboard"}."File" ("目标"), "Path"=w497, "Hide Grid"=TRUE ("始终覆盖")) -> (error out=w496:errorcluster)  [unwired: 2 in, 6 out]
            n267 = call <vilib>:"Application Directory.vi"() -> ("Application Directory"=w490:path)
            n268 = case shown="1" "Mode Selection" {
              tunnel: [w504 w507] -> w493
              tunnel: w496 -> [w505 w506]
              frame 0, Default {
                n269 = script code="%%   图像动态处理\n%-----------------\n%通过此函数得到页面高度；\n%function [h_real,u,u2,time1]=sep_fun()  %函数命名\n%tic;\n%% 1 --------------------\n%-------------------------获取图像；\n%time=VI;   %运行VI得到获取的图像和时间“time”\n%clear;\n%clc;\nu=imread('C:\\Program Files\\北控\\data\\Tem.bmp');  %读取图像\n%% -------2.1 辨识区域选择\n%imshow(u)\n[M,N,P]=size(u);      %M,N为矩阵的行列；M为图像高度，N为图像长度；\n%break\nbei1=8;            %间隔16个像素扫描；\nbei=round(N./bei1);          %bei为粗化倍数\nA=zeros(1,bei);     %初始化向量A，将其作为每列的平均值；\nfor i=1:bei;\nA(i)=round(sum(u(:,i*bei1))./M); %每列平均后取整数；   注意8\nend\nx2=max(A); x1=min(A); y1=x2-x1;\nfor i=1:bei;  %将A1归一化；\n  A(i)=round(255*(A(i)-x1)/y1);\nend\n\n%% ---2.2 确定区域内小于40的值，既是找出黑色区域；\nB=zeros(1,bei);    \nfor i=1:bei\n   if A(i)<=40;  %设定黑色区域的区分值；\n       B(i)=1;   %小于80记点  为1     \n   else\n       B(i)=0;   %大于80记点  为0\n   end\nend\n\n%% 2.3---找出连续为黑色，突然为白色的点，并进行标记\nfor i=1:bei-1    \n    B(i+1)=B(i)+B(i+1); %B为标记点的累加值\n    j=i+1;              %记下除以倍数后的坐标；\n    if B(i+1)>0 & B(i+1)==B(i) %B>0而且不再增加，说明搜索到达视窗区域；     \n        break \n    end        \nend\nk=j+1; k=(k+1.75)*bei1;  %k为视窗右边；\nj=(j-1).*bei1;         %j为视窗左边；\n\nu1=u(:,j:k) ;     %令u1为截取分析区域的矩阵；\n%imshow(u1)\n\n%% %--------2.4 对截取区域图进行分析\n[M1,N1]=size(u1);      %M,N为矩阵的行列；M为图像高度，N为图像长度；\nA1=zeros(M1,1);     %初始化向量A，将其作为每列的平均值；\nfor i=1:M1;\nA1(i)=round(sum(u1(i,:))./N1); %每行平均后取整数；   注意8\nend\n\n%% ----2.5.1 从下往上搜索分离边界。\nfor i=1:max(size(A1));\n    A2(i)=A1(max(size(A1))-i+1); %将A1转换方向变为A2；\nend\n\n\n%---记录A2中大于150点的地址。\nfor i=1:max(size(A1));\n    if A2(i)<=60;      %   ？？？？？？？？？？？？？\n        k1=i;\n    else\n        break\n    end    \nend\nk1=M1-k1;  j1=k1-895;\n%k1=k1-100;  j1=j1+100;\nu2=u1(j1:k1,:);\n%% ---对视窗区域进行辨识\nfor i=1:k1-j1;\n    A3(i)=round(sum(u2(i,:))./(k-j)); %每行平均后取整数；   注意8\nend\nx2=max(A3); x1=min(A3); y1=x2-x1;\nfor i=1:k1-j1;  %将A1归一化；\n  A3(i)=round(255*(A3(i)-x1)/y1);\nend\n\n%p=round((j+k)./2);\n%A2=A1(j:k);  %框选出来的均值\n%C=zeros(p,1); %差值的空向量\ncaiyang=10;    %设定采样间隔；\np=caiyang;\n%% 2.4.1 开始从中间往上计算差值；\nfor i=1:max(size(A3))-p\n   C(i)=abs(A3(i+p)-A3(i)); %框选出来的差值，每间隔5个像素计算差值；\nend\n[q,h1]=max(C);      % 第一种正常判断突变最大点   h为相对坐标\n%[q,h2]=min(A3);    % 第二种用及值判断区域最黑点   h1 为相对坐标\n\n\n\n%if h1<p & h1<100 & h1>k1-100;  %如果判断的点在有效区域外，用第二种\n %   h=h2+j1;                   %则绝对坐标为\n%else     %如果在区域内\n\n%% 对油水界面进行细分\n%A4=A3(h1-p:h1+p);    %细分变量\n%[gray,adr]=max(A4);\n%h=j1+h1-p+adr;    %得到准确的油水分离像素点；\nh=j1+h1;    %得到准确的油水分离像素点；\n%end\n\n\n\n%% 对油水界面进行计算，并将“h”转化为距离视窗底面的高度\nadjust=1;\narea=0.444;\nt=adjust.*133./(k1-j1);  %每个像素的长度；\n%h_rela=M-h;            %将h转化为距离端盖下端的距离 的像素点；\nh_rela=k1-h;\nh_real=h_rela.*t;     %将h转化为距离端盖下端的实际距离；\n\nu(h-1:h+1,:)=0;  % 将整体图片u的分离界面涂黑;\nimshow(u); % 绘制整体图形u;\nfid=fopen('C:\\Program Files\\北控\\data\\H_temp.txt','w');       %h为液面高度值；\nfprintf(fid,'%f\\n',h_real);        %%%q为你要写入的数据，“'%f”为数据格式\nfclose(fid);"("??"=w505) -> ("??"=w504:errorcluster)
              }
              frame 1 {
                n270 = script code="%%   图像动态处理\n%-----------------\n%通过此函数得到页面高度；\n%function [h_real,u,u2,time1]=sep_fun()  %函数命名\n%tic;\n%% 1 --------------------\n%-------------------------获取图像；\n%time=VI;   %运行VI得到获取的图像和时间“time”\n%clear;\n%clc;\nu=imread('C:\\Program Files\\北控\\data\\Tem.bmp');  %读取图像\n%% -------2.1 辨识区域选择\n%imshow(u)\n[M,N,P]=size(u);      %M,N为矩阵的行列；M为图像高度，N为图像长度；\n%break\nbei1=8;            %间隔16个像素扫描；\nbei=round(N./bei1);          %bei为粗化倍数\nA=zeros(1,bei);     %初始化向量A，将其作为每列的平均值；\nfor i=1:bei;\nA(i)=round(sum(u(:,i*bei1))./M); %每列平均后取整数；   注意8\nend\nx2=max(A); x1=min(A); y1=x2-x1;\nfor i=1:bei;  %将A1归一化；\n  A(i)=round(255*(A(i)-x1)/y1);\nend\n\n%% ---2.2 确定区域内小于40的值，既是找出黑色区域；\nB=zeros(1,bei);    \nfor i=1:bei\n   if A(i)<=40;  %设定黑色区域的区分值；\n       B(i)=1;   %小于80记点  为1     \n   else\n       B(i)=0;   %大于80记点  为0\n   end\nend\n\n%% 2.3---找出连续为黑色，突然为白色的点，并进行标记\nfor i=1:bei-1    \n    B(i+1)=B(i)+B(i+1); %B为标记点的累加值\n    j=i+1;              %记下除以倍数后的坐标；\n    if B(i+1)>0 & B(i+1)==B(i) %B>0而且不再增加，说明搜索到达视窗区域；     \n        break \n    end        \nend\nk=j+1; k=(k+1.75)*bei1;  %k为视窗右边；\nj=(j-1).*bei1;         %j为视窗左边；\n\nu1=u(:,j:k) ;     %令u1为截取分析区域的矩阵；\n%imshow(u1)\n\n%% %--------2.4 对截取区域图进行分析\n[M1,N1]=size(u1);      %M,N为矩阵的行列；M为图像高度，N为图像长度；\nA1=zeros(M1,1);     %初始化向量A，将其作为每列的平均值；\nfor i=1:M1;\nA1(i)=round(sum(u1(i,:))./N1); %每行平均后取整数；   注意8\nend\n\n%% ----2.5.1 从下往上搜索分离边界。\n%for i=1:max(size(A1));\n%    A2(i)=A1(max(size(A1))-i+1); %将A1转换方向变为A2；\n% end\n\n\n%---记录A2中大于150点的地址。\nfor i=1:max(size(A1));\n    if A1(i)<=60;      %   ？？？？？？？？？？？？？\n        j1=i;\n    else\n        break\n    end    \nend\n%k1=M1-k1;  \nk1=j1+895;\nu2=u1(j1:k1,:);\n%break\n%% ---对视窗区域进行辨识\nfor i=1:k1-j1;\n    A3(i)=round(sum(u2(i,:))./(k-j)); %每行平均后取整数；   注意8\nend\nx2=max(A3); x1=min(A3); y1=x2-x1;\nfor i=1:k1-j1;  %将A1归一化；\n  A3(i)=round(255*(A3(i)-x1)/y1);\nend\n\n%p=round((j+k)./2);\n%A2=A1(j:k);  %框选出来的均值\n%C=zeros(p,1); %差值的空向量\ncaiyang=10;    %设定采样间隔；\np=caiyang;\n%% 2.4.1 开始从中间往上计算差值；\nfor i=1:max(size(A3))-p\n   C(i)=abs(A3(i+p)-A3(i)); %框选出来的差值，每间隔5个像素计算差值；\nend\n[q,h1]=max(C);      % 第一种正常判断突变最大点   h为相对坐标\n%[q,h2]=min(A3);    % 第二种用及值判断区域最黑点   h1 为相对坐标\n\n\n\n%if h1<p & h1<100 & h1>k1-100;  %如果判断的点在有效区域外，用第二种\n %   h=h2+j1;                   %则绝对坐标为\n%else     %如果在区域内\n\n%% 对油水界面进行细分\n%A4=A3(h1-p:h1+p);    %细分变量\n%[gray,adr]=max(A4);\n%h=j1+h1-p+adr;    %得到准确的油水分离像素点；\nh=j1+h1;    %得到准确的油水分离像素点；\n%end\n\n\n\n%% 对油水界面进行计算，并将“h”转化为距离视窗底面的高度\nadjust=1;\narea=0.444;\nt=adjust.*133./(k1-j1);  %每个像素的长度；\n%h_rela=M-h;            %将h转化为距离端盖下端的距离 的像素点；\nh_rela=k1-h;\nh_real=h_rela.*t;     %将h转化为距离端盖下端的实际距离；\n\nu(h-1:h+1,:)=0;  % 将整体图片u的分离界面涂黑;\nimshow(u); % 绘制整体图形u;\nfid=fopen('C:\\Program Files\\北控\\data\\H_temp.txt','w');       %h为液面高度值；\nfprintf(fid,'%f\\n',h_real);        %%%q为你要写入的数据，“'%f”为数据格式\nfclose(fid);"("??"=w506) -> ("??"=w507:errorcluster)
              }
            }
            n271 = Path To String(path=w490) -> (string=w489:string)
            n272 = Concatenate Strings(w489, "\\data\\H_temp.txt" ("字符串")) -> (w487:string)
            n273 = String To Path(string=w487) -> (path=w491:path)
            n274 = local read "WaterValueCal"() -> (w474:bool)
            n275 = Read from Text File(file (use dialog)=w491, error in=w493) -> (text=w492:string, error out=w501:errorcluster)  [unwired: 2 in, 2 out]
            n276 = local read "OilValueCal"() -> (w479:bool)
            n277 = case shown="无错误" w501 {
              frame No Error {
              }
              frame Error {
              }
            }
            n278 = Fract/Exp String To Number(string=w492) -> (number=w476:dbl)  [unwired: 3 in, 1 out]
            n279 = call "Oil.vi"("Adjust"="Adjust", "循环次数"=w503, "PreValue"="PreWaterValue", "ValueCal"=w474, "当前值"="WaterSeperation1.0", "Seperation1.0"=w476) -> ("OilValue1"=w471:dbl)  [unwired: 5 in]
            "WaterValue" <- w471
            n280 = call "Oil.vi"("Adjust"="Adjust", "循环次数"=w503, "PreValue"="PreOilValue", "ValueCal"=w479, "当前值"=w476, "Seperation1.0"="OilSeperation1.0") -> ("OilValue1"=w477:dbl)  [unwired: 5 in]
            "OilValue" <- w477
            n281 = local write "PreWaterValue"(w471) -> ()
            n282 = local write "PreOilValue"(w477) -> ()
          }
          frame #4 {
            # "ISCO泵 相关值读取"
            n283 = local read "ISCOTCP"() -> (w525:refnum<k5>)
            n284 = call "ReadDate.vi"("18000IN"=w525) -> ("18000OUT"=w524:dbl[])  [unwired: 8 in, 2 out]
            n285 = Index Array(array=w524, index #1=0 ("索引"), index #2=1 ("索引"), index #3=2 ("索引"), index #4=3 ("索引"), index #5=4 ("索引"), index #6=5 ("索引"), index #7=6 ("索引"), index #8=7 ("索引")) -> (element #1=→"Flow Rate A":dbl, element #2=→"Pressure A":dbl, element #3=→"Flow Setpoint A":dbl, element #4=→"Pressure Setpoint A":dbl, element #5=→"Flow Rate B":dbl, element #6=→"Pressure B":dbl, element #7=→"Flow Setpoint B":dbl, element #8=→"Pressure Setpoint B":dbl)
          }
          frame #5 {
            # "圧力 压差曲线 画线"
            n286 = local read "文本下拉列表"() -> (w531:u16)
            n287 = local read "数值输入控件"() -> (w530:dbl)
            n288 = case shown="0, 默认" w531 {
              tunnel: w530 -> [w538 w541]
              tunnel: [w538 w539] -> w526
              frame 0, Default {
              }
              frame 1 {
                n289 = Multiply(x=w541, y=60.0) -> (x*y=w539:dbl)
              }
            }
            n290 = Quotient & Remainder(x=w529, y=w526) -> (x-y*floor(x/y)=w528:dbl)  [unwired: 1 out]
            n291 = Equal To 0?(x=w528) -> (x = 0?=w527:bool)
            n292 = case shown="真" w527 {
              tunnel: w526 -> [_ w532]
              frame False {
              }
              frame True {
                n293 = stacked-sequence {
                  tunnel: w532 -> [w533 _ _]
                  frame #0 {
                    n294 = property on="压力曲线" class="WFChart (严格)"("XScale.Multiplier"=w533) -> ()  [unwired: 2 in, 2 out]
                    n295 = property on="压差曲线" class="WFChart (严格)"("XScale.Multiplier"=w533) -> ()  [unwired: 2 in, 2 out]
                  }
                  frame #1 {
                    n296 = local read "P1(夹持器前端)"() -> (w536:dbl)
                    n297 = local read "P2(夹持器后端)"() -> (w535:dbl)
                    n298 = Bundle("P1(夹持器前端)"=w536, "P2(夹持器后端)"=w535) -> (→"压力曲线":cluster{"P1(夹持器前端)":dbl, "P2(夹持器后端)":dbl})  [unwired: 1 in]
                  }
                  frame #2 {
                    n299 = local read "DIF1"() -> (→"压差曲线":dbl)
                  }
                }
              }
            }
          }
        }
        n300 = local read "btnExit"() -> (w292:bool)
      }
      n301 = while {
        tunnel: [w544] -> _
        stop <- "btnExit" stop-if-true
        n302 = local read "StartSaving"() -> (w542:bool)
        n303 = local write "Stop"(0.0 ("Stop")) -> ()
        n304 = local write "Suspend"(0.0 ("Suspend")) -> ()
        n305 = Wait Until Next ms Multiple(millisecond multiple=u32 100 ("毫秒计时值")) -> ()  [unwired: 1 out]
        n306 = case shown="真" w542 {
          tunnel: [w548 w549] -> w544
          frame False {
            n307 = local read "DataBase"() -> (w548:T5)
          }
          frame True {
            n308 = Get Date/Time In Seconds() -> (seconds since 1Jan1904=w551:timestamp)
            n309 = while {
              tunnel: w551 -> [w570]
              tunnel: [w572] -> w549
              shift-right: [w561] -> _
              shift-left: 0.0 -> [w562]
              i -> [w558]
              stop <- w573 stop-if-true
              n310 = local read "Stop"() -> (w574:dbl)
              n311 = Get Date/Time In Seconds() -> (seconds since 1Jan1904=w571:timestamp)
              n312 = Wait (ms)(milliseconds to wait=u32 1000 ("等待时间（毫秒）")) -> ()  [unwired: 1 out]
              n313 = Subtract(x=w571, y=w570) -> (x-y=w569:dbl)
              n314 = case shown="1" "文本下拉列表" {
                tunnel: w558 -> [w611 w616]
                tunnel: [w610 w615] -> w554
                tunnel: "数值输入控件" -> [w609 w614]
                frame 0, Default {
                  n315 = Quotient & Remainder(x=w611, y=w609) -> (x-y*floor(x/y)=w610:dbl)  [unwired: 1 out]
                }
                frame 1 {
                  n316 = Multiply(x=w614, y=60) -> (x*y=w612:dbl)
                  n317 = Quotient & Remainder(x=w616, y=w612) -> (x-y*floor(x/y)=w615:dbl)  [unwired: 1 out]
                }
              }
              n318 = Equal?(x=w574, y=1.0) -> (x = y?=w573:bool)
              n319 = Quotient & Remainder(x=w569, y=3600) -> (x-y*floor(x/y)=w566:dbl, floor(x/y)=→"h":dbl)
              n320 = local read "Suspend"() -> (w555:dbl)
              n321 = Equal To 0?(x=w555) -> (x = 0?=w553:bool)
              n322 = Equal To 0?(x=w554) -> (x = 0?=w552:bool)
              n323 = Quotient & Remainder(x=w566, y=60.0) -> (x-y*floor(x/y)=→"s":dbl, floor(x/y)=→"m":dbl)
              n324 = And(x=w553, y=w552) -> (x .and. y?=w557:bool)
              n325 = local read "DataBase"() -> (w560:T5)
              n326 = case shown="真" w557 {
                tunnel: w560 -> [w587 w607]
                tunnel: [w604 w607] -> w572
                tunnel: w562 -> [w603 w608]
                tunnel: [w602 w608] -> w561
                frame True {
                  n327 = Increment(x=w603) -> (x+1=w602:dbl)
                  "Number" <- w602
                  n328 = local read "Pressure Setpoint A"() -> (w584:dbl)
                  n329 = local read "Pressure Setpoint B"() -> (w580:dbl)
                  n330 = local read "Flow Setpoint A"() -> (w585:dbl)
                  n331 = local read "Flow Setpoint B"() -> (w581:dbl)
                  n332 = local read "OuterPre(MPa)"() -> (w592:dbl)
                  n333 = local read "TracePre(MPa)"() -> (w591:dbl)
                  n334 = local read "CurrentVol(ml)"() -> (w590:dbl)
                  n335 = local read "InnerPre(MPa)"() -> (w589:dbl)
                  n336 = local read "P1(夹持器前端)"() -> (w594:dbl)
                  n337 = local read "P2(夹持器后端)"() -> (w593:dbl)
                  n338 = Get Date/Time String ("获取日期/时间字符串")(want seconds? (F)=TRUE ("需要秒？(F)")) -> (date string=w606:string, time string=w601:string)  [unwired: 2 in]
                  n339 = local read "WaterValue"() -> (w588:dbl)
                  n340 = local read "Flow Rate A"() -> (w583:dbl)
                  n341 = local read "Flow Rate B"() -> (w579:dbl)
                  n342 = call <vilib>:"Space Constant.vi"() -> ("String"=w600:string)
                  n343 = local read "Pressure A"() -> (w582:dbl)
                  n344 = local read "Pressure B"() -> (w578:dbl)
                  n345 = local read "OilValue"() -> (w597:dbl)
                  n346 = local read "Weight"() -> (w596:dbl)
                  n347 = Concatenate Strings(w606, w600, w601) -> (w598:string)
                  n348 = local read "DIF1"() -> (w595:dbl)
                  n349 = Bundle(w598, "OilValue"=w597, "WaterValue"=w588, "Weight"=w596, "DIF1"=w595, "P1(夹持器前端)"=w594, "P2(夹持器后端)"=w593, "OuterPre(MPa)"=w592, "TracePre(MPa)"=w591, "CurrentVol(ml)"=w590, "InnerPre(MPa)"=w589, "Flow Setpoint A"=w585, "Pressure Setpoint A"=w584, "Flow Rate A"=w583, "Pressure A"=w582, "Flow Setpoint B"=w581, "Pressure Setpoint B"=w580, "Flow Rate B"=w579, "Pressure B"=w578) -> (w605:T9)  [unwired: 1 in]
                  n350 = local read "数据库文件名"() -> (w586:string)
                  n351 = call <vilib>:"DB Tools Insert Data.vi"("data"=w605, "columns"=string[] ["RecordingTime", "CumulativeOilProduction", "CumulativeWaterProduction", "BalanceValue", "DifferencialPressure", "Pressure1", "Pressure2", "CPPOuterPre", "CPPTracePre", "CPPCurrentVol", "CPPInnerPre", "FlowSetpointA", "PressureSetpointA", "FlowRateA", "PressuerA", "FlowSetpointB", "PressureSetpointB", "FlowRateB", "PressuerB"], "table"=w586, "connection reference"=w587) -> ("connection reference out"=w604:T5)  [unwired: 6 in, 1 out]
                }
                frame False {
                }
              }
            }
          }
        }
      }
      n352 = disable-structure shown="禁用" {
        disable-tunnel: w278 -> [w284 _]
        frame Disabled {
          n353 = property class="IICImagingControl"(reference=w284) -> (reference out=w282:refnum<k7>, error out=w281:errorcluster, "LiveVideoRunning"=w283:bool)  [unwired: 1 in]
          n354 = case shown="假" w283 {
            tunnel: w282 -> [_ w288]
            tunnel: w281 -> [w285 w287]
            tunnel: [w285 w286] -> w280
            frame False {
            }
            frame True {
              n355 = invoke class="IICImagingControl" method="LiveStop"(reference=w288, error in=w287) -> (error out=w286:errorcluster)  [unwired: 1 in, 2 out]
            }
          }
          n356 = case shown="无错误" w280 {
            frame No Error {
            }
            frame Error {
            }
          }
        }
        frame Enabled {
        }
      }
      n357 = TCP Close Connection(connection ID=w279) -> (error out=w277:errorcluster)  [unwired: 2 in, 1 out]
      n358 = case shown="无错误" w277 {
        frame No Error {
        }
        frame Error {
        }
      }
    }
  }
